vi "BeamScanner.vi"() -> ()   [LabVIEW 2016]
uses:
  C:/Program Files/Ocean Optics/OmniDriver/OOI_HOME/NETOmniDriver-NET40.dll
  Program Files/Ocean Optics/OmniDriver/OOI_HOME/NETOmniDriver-NET40.dll
  <vilib>/DAQmx/write.llb/DAQmx Write (Digital Bool 1Line 1Point).vi
  <vilib>/DAQmx/write.llb/DAQmx Write (Analog DBL 1Chan 1Samp).vi
  <vilib>/DAQmx/write.llb/DAQmx Write (Analog 1D DBL NChan 1Samp).vi
  <vilib>/DAQmx/write.llb/DAQmx Write (Analog 2D DBL NChan NSamp).vi
  <vilib>/Analysis/baseanly.llb/Mean (DBL).vi
  <vilib>/DAQmx/read.llb/DAQmx Read (Raw 1D I16).vi
  <vilib>/Analysis/1siggen.llb/Ramp Pattern by Samples.vi
  <vilib>/DAQmx/create/channels.llb/DAQmx Create Channel (DO-Digital Output).vi
  <vilib>/DAQmx/miscellaneous.llb/DAQmx Fill In Error Info.vi
  <vilib>/DAQmx/create/channels.llb/DAQmx Create Channel (AO-Voltage-Basic).vi
  resources/MotorPosition.vi
  <vilib>/DAQmx/create/channels.llb/DAQmx Create Channel (AI-Voltage-Basic).vi
  <vilib>/DAQmx/configure/timing.llb/DAQmx Timing (Sample Clock).vi
  <vilib>/DAQmx/configure/trigger.llb/DAQmx Start Trigger (Digital Edge).vi
  OCM/private/global.vi
  resources/xy_stack_global.vi
  <vilib>/Analysis/NI_AALBase.lvlib
  <resource>/objmgr/daqmx.rc
panel:
  out "Laser Blocking":string
  in  "Background":bool
  out "floor(x/y)":i32
  in  "Scan no.":i32
  in  "XY-Stack setup":bool
  in  "xy-Stacking":bool
  out "OCM Settings":T1
  out "Processed FFT":cluster{dbl[], "X":dbl[]}(graph)
  in  "length":i32=50
  in  "FFT index":i32=10
  out "OCM Array":dbl[][][](array[numeric])
  out "error out 2":errorcluster
  out "error out":errorcluster
  in  "OCM Setup":bool
  in  "Home X":dbl=-115.0
  in  "Home  Y":dbl=-88.0
  in  "sampling rate (ADC)":u32(ring)=1250000 items=["500000"=500000, "750000"=750000, "1000000"=1000000, "1250000"=1250000]
  in  "Intgration time [us]":u32=44444 min=100 max=10000000 step=1
  in  "Wavelength max":dbl=761.0 min=200.0 max=1100.0 step=1.0
  in  "Wavelength min":dbl=374.0 min=200.0 max=1100.0 step=1.0 format="%#.4g"
  out "spectral image":u32[][][](array[numeric])
  out "read task":refnum<k21>
  out "write task":refnum<k21>
  in  "Detector":u16(ring) items=["PMT", "QEPro", "Basler OCM", "Basler Confocal"]
  out "scanning waveforms":dbl[][](array[numeric])
  out "Retrace":dbl[][](array[numeric])
  in  "Move to z":bool
  out "z-Position":sgl format="%.2g"
  out "xy-Position [µm]":sgl[](array[numeric]) min=0 max=500
  in  "Thrown samples":i16=500
  in  "Throw away":bool
  out "Samples/Pixel":u32
  in  "PMT output range":dbl(ring)=0.1 items=["-0,1V – 0,1V"=0.1, "-0,2V – 0,2V"=0.2, "-0,5V – 0,5V"=0.5, "-1V – 1V"=1.0, "-2V – 2V"=2.0, "-5V – 5V"=5.0, "-10V – 10V"=10.0]
  out "Time of last scan memory":string
  out "Info File contents memory":string
  out "Info File contents":string
  out "Time per line [s]":dbl format="%#.1g"
  out "Time of last scan":string
  out "scaling factor (length/voltage)":dbl=228.9
  in  "Additional info":string
  in  "Save":bool
  in  "Quit":bool
  in  "PMT sensitivity":dbl min=-1989.12 max=1989.12 format="%#.2f"
  in  "requested z-Position":dbl min=0.0 max=10.0
  in  "# steps":u16=20 step=1 format="%#.0f"
  out "Duration (m.s)":string
  in  "Scanrate (pixels/s)":u32(ring)=10000 items=["250 kHz"=250000, "125 kHz"=125000, "50 kHz (!)"=50000, "25 kHz (!)"=25000, "10 kHz (?)"=10000, "5 kHz (?)"=5000, "2 kHz"=2000, "1 kHz"=1000, "500 Hz"=500, "200 Hz"=200, "100 Hz"=100]
  out "Optimal":string
  out "Optimal pixel size [nm]":dbl format="%#.0f"
  in  "NA":dbl=1.0 min=0.0
  in  "Swap Memory":bool
  out "Memory":dbl[][](graph)
  out "System":bool
  in  "Use white point":bool
  in  "Magnification":dbl=20.0
  in  "Go home":bool
  in  "Go to white point":bool
  in  "z-Maximum val":dbl min=0.0 max=500.0 format="%#.2f"
  in  "z-Minimum val":dbl min=0.0 max=500.0 format="%#.2f"
  in  "z-Stacking":bool
  in  "Step size":dbl=1.0 min=0.0
  in  "z-Minimum":dbl(slide) min=0.0 max=500.0 step=1.0 scale=0.0..500.0
  in  "z-Maximum":dbl(slide)=0.30612244897959184 min=370.0 max=500.0 step=1.0 scale=0.0..500.0
  out "Path":path
  in  "File identifier":string="unnamed_file"
  in  "Save Image":bool
  in  "Scan":bool
  in  "y-Offset":dbl=-160.0 min=-448.0 max=448.0 format="%#.2f"
  in  "x-Offset":dbl=-220.0 min=-448.0 max=448.0 format="%#.2f"
  in  "Field of View":dbl(ring)=0.471281296023564 items=["4x4 µm"=0.01747106355099367, "8x8 µm"=0.03494212710198734, "16x16 µm"=0.06988425420397468, "32x32 µm"=0.13976850840794935, "64x64 µm"=0.2795370168158987, "128x128 µm"=0.5590740336317974, "256x256 µm"=1.1181480672635948, "512x512 µm"=2.2362961345271897, "1024x1024 µm"=4.472592269054379, "0x0"=0.0]
  out "Image":dbl[][](graph)
  in  "Number of pixels":i32(ring)=128 items=["8x8"=8, "16x16"=16, "32x32"=32, "64x64"=64, "128x128"=128, "256x256"=256, "512x512"=512, "1024x1024"=1024, "optimal"=1280]
  # "OCM debugging"
  # "make setup button"
  # "MIN 7000 for QEPro"
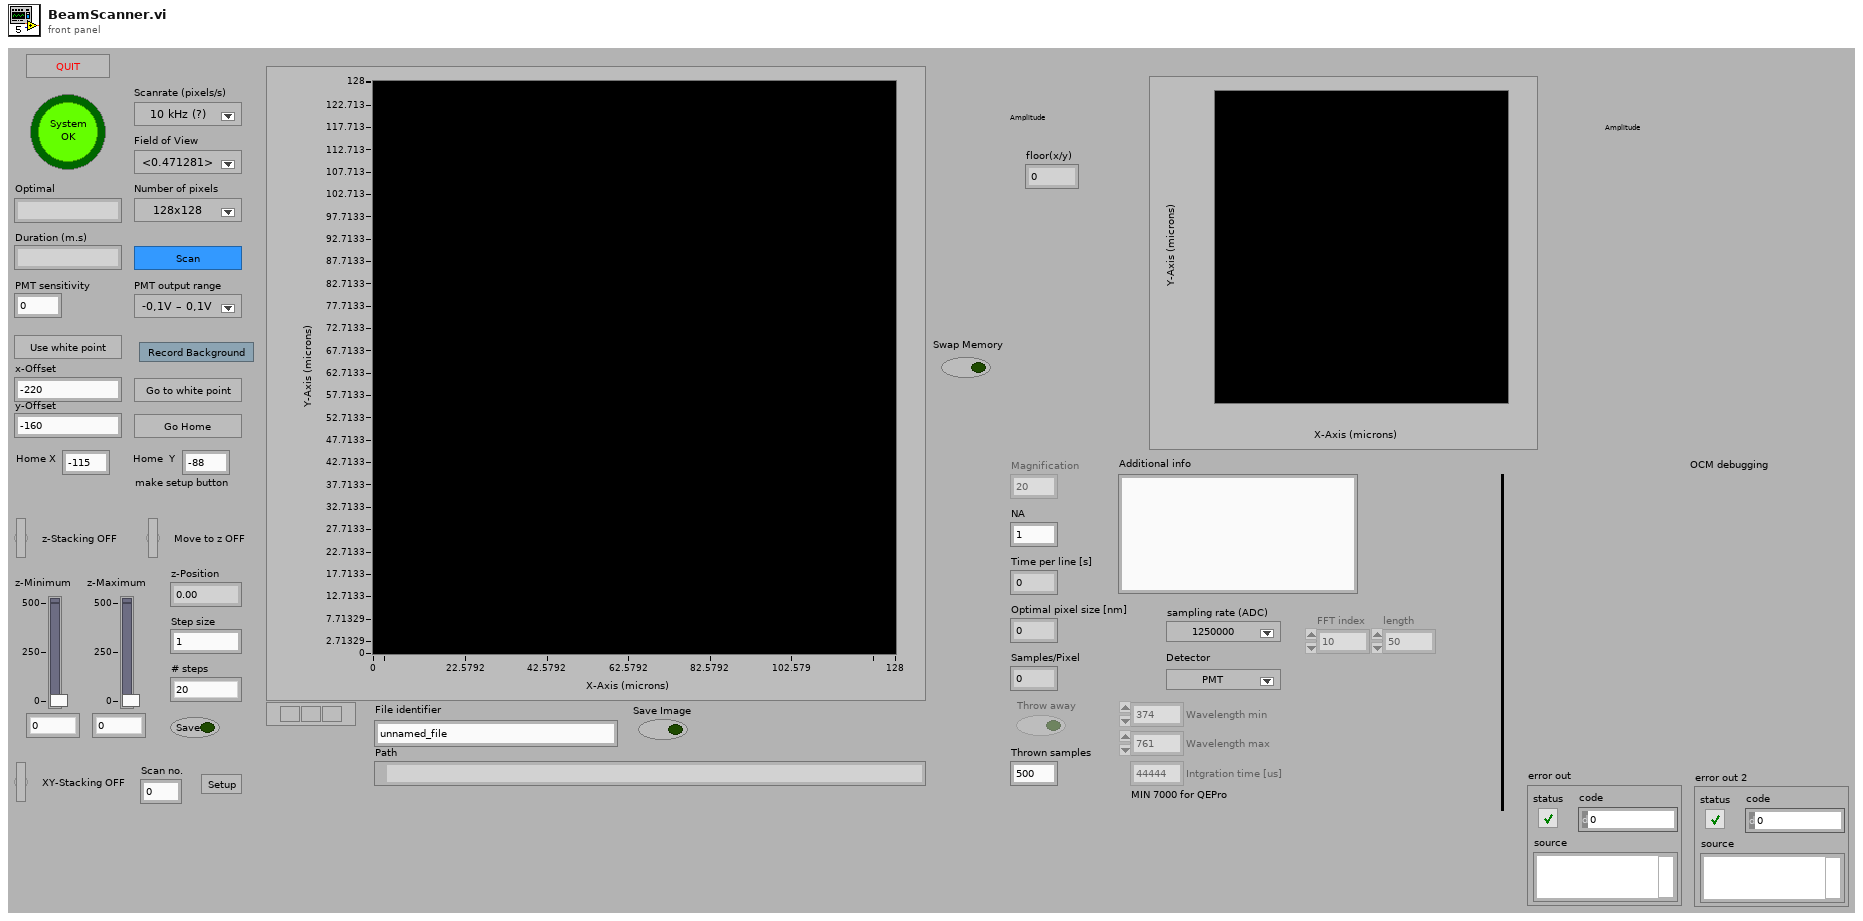
[diagram p1: front panel]
types:
  T1 = cluster{"Binning be4 FFT ":bool, "Pixels FFT":i32, "Camera averaging":bool, "FFT averaging":bool, "FFT AVG Size":dbl, "BG subtraction":bool, "DC compensation":bool, "BG Array":dbl[], "DC Array":dbl[], "k-array":dbl[], "axial distance array":dbl[], "k-ramp":dbl[]}
  T2 = enum8{"Enabled", "Disabled", "Disabled and Grayed Out"}
  T3 = enum32{"Invalid", "Standard", "Closed", "Hidden", "Minimized", "Maximized"}
  T4 = typedef "LVStringsAndValuesArrayTypeDef_DBL.ctl" = cluster{"String":string, "Value":dbl}[]
  T5 = typedef "LVStringsAndValuesArrayTypeDef_I32.ctl" = cluster{"String":string, "Value":i32}[]
  T6 = typedef "LVOffsetAndMultiplierTypeDef.ctl" = cluster{"Offset":dbl, "Multiplier":dbl}
  T7 = typedef "Maya2000 basic info.ctl" = cluster{"This instruments index":i32, "Name+SerialNumber":string, "Number Dark pixels":i32, "NumberOfPixels\nper spectrum":i32, "NumberOf Maya2000 instrm.":i32, "MaximumIntegrationTime\n[us]":i32, "MinimumIntegrationTime\n[us]":i32}
  T8 = typedef "IMAQ Image.ctl" = refnum<image>
  T9 = cluster{"Ramp Pattern":dbl[], "FFT Processed":dbl[]}
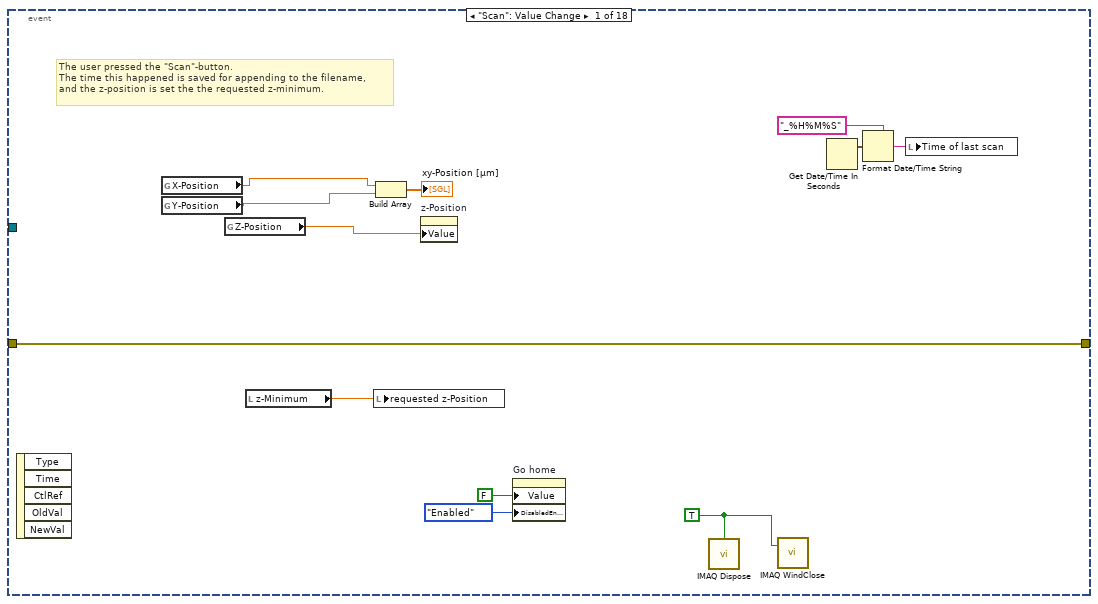
[diagram p3: hidden frame]
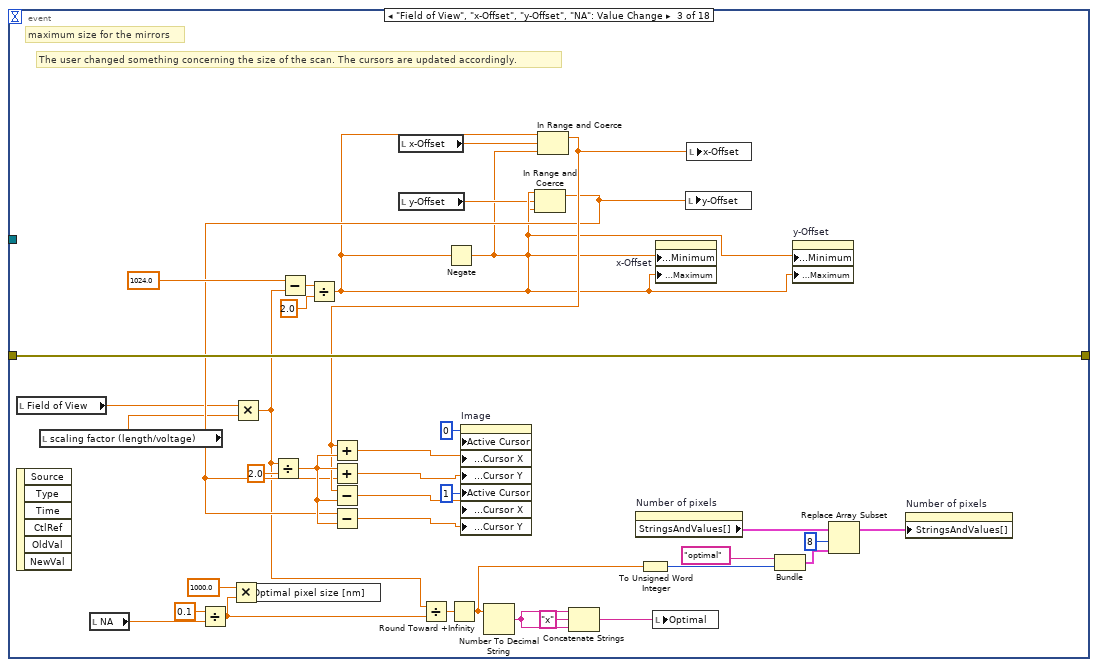
[diagram p5: hidden frame]
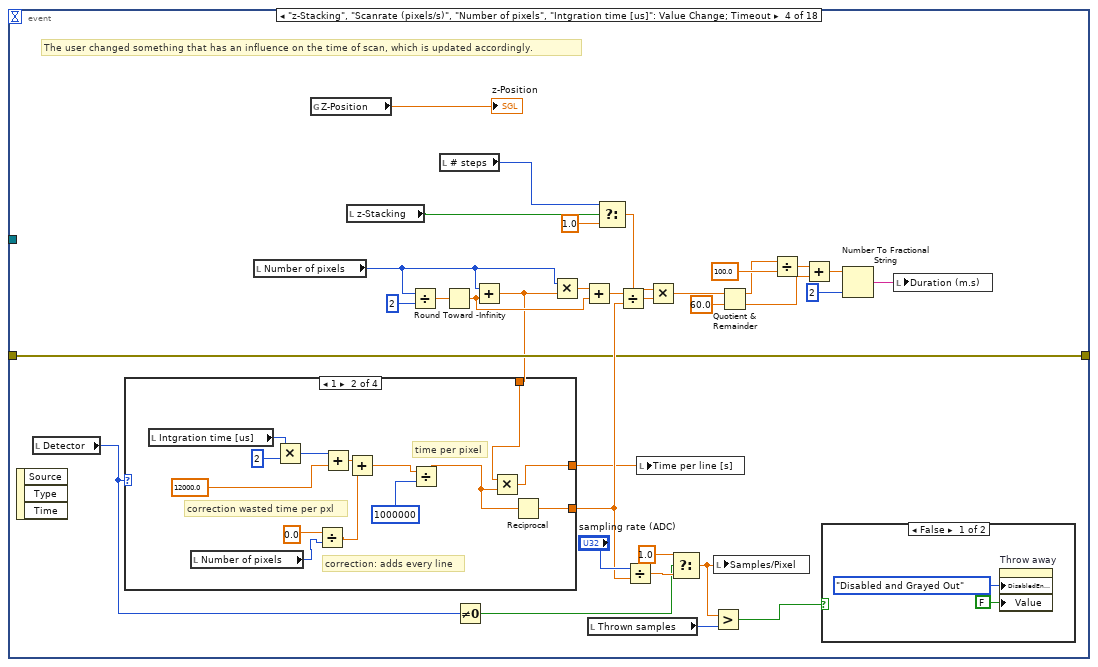
[diagram p6: hidden frame]
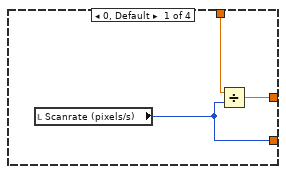
[diagram p7: hidden frame]
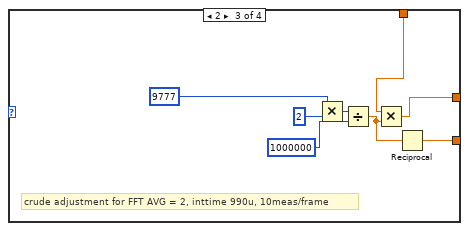
[diagram p8: hidden frame]
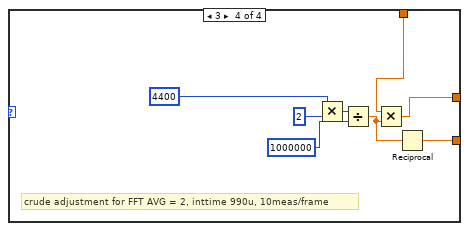
[diagram p9: hidden frame]
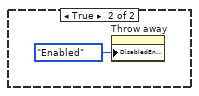
[diagram p10: hidden frame]
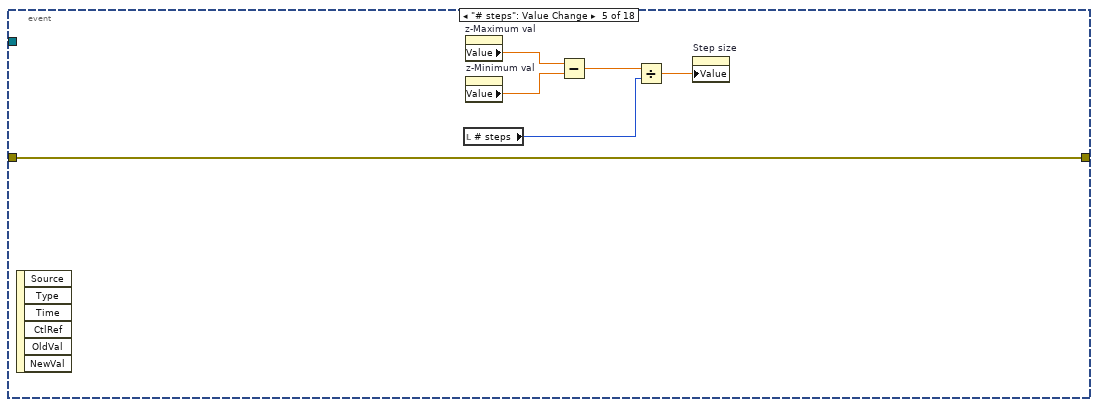
[diagram p11: hidden frame]
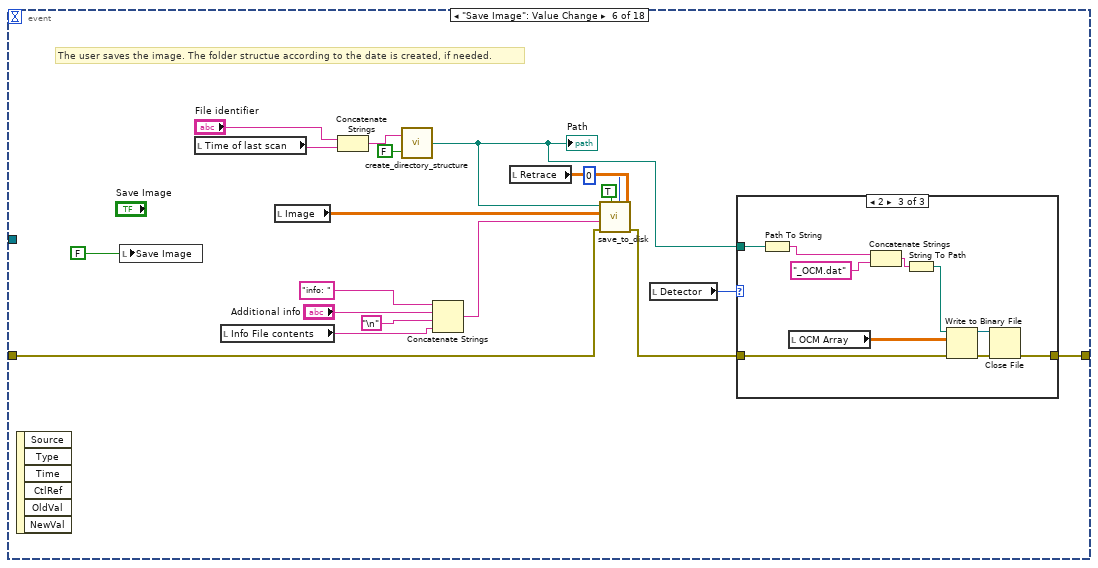
[diagram p12: hidden frame]
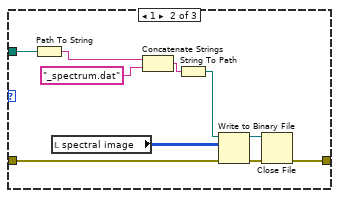
[diagram p14: hidden frame]
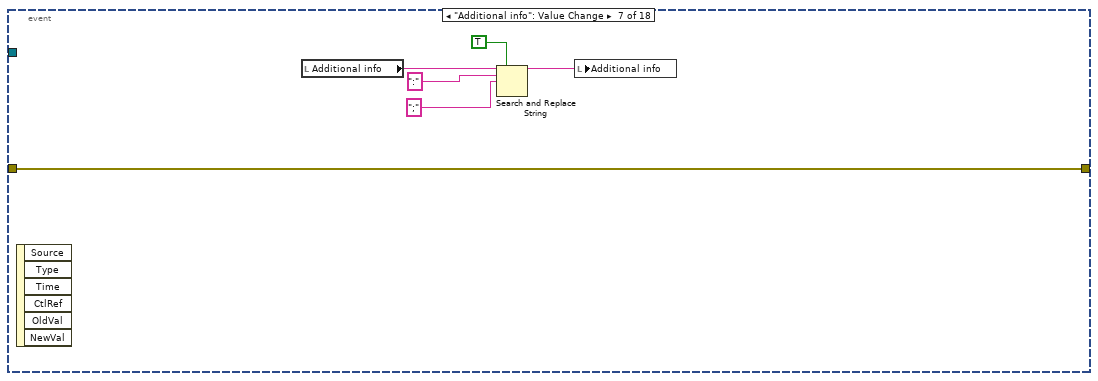
[diagram p15: hidden frame]
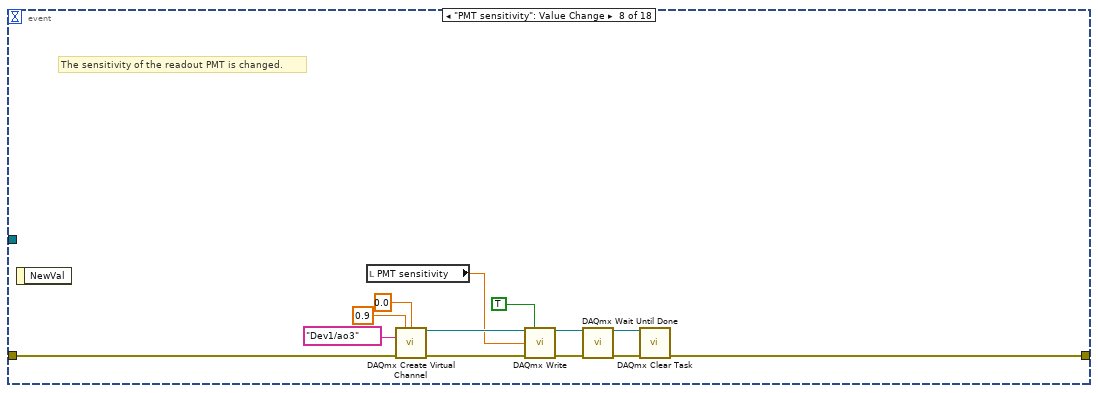
[diagram p16: hidden frame]
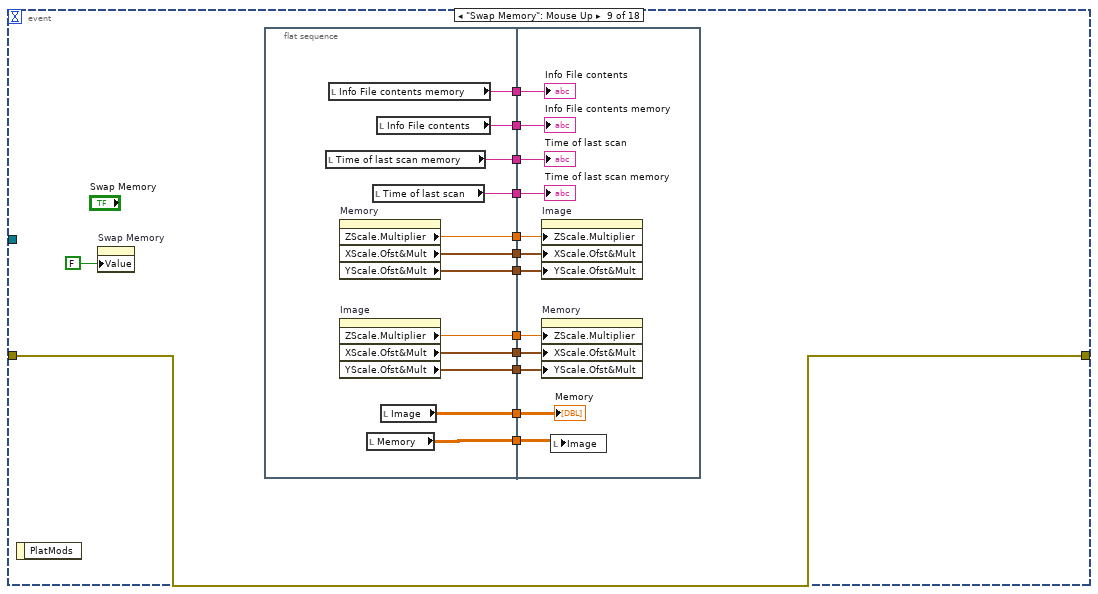
[diagram p17: hidden frame]
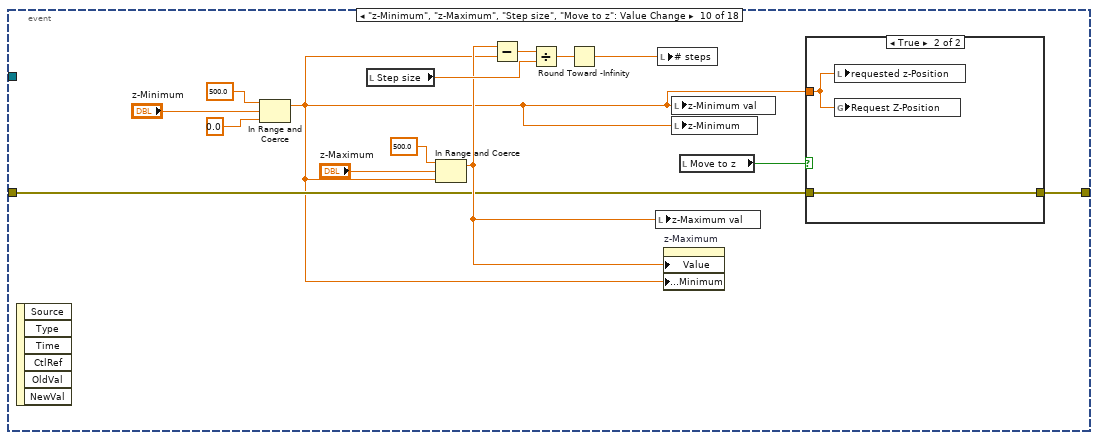
[diagram p18: hidden frame]
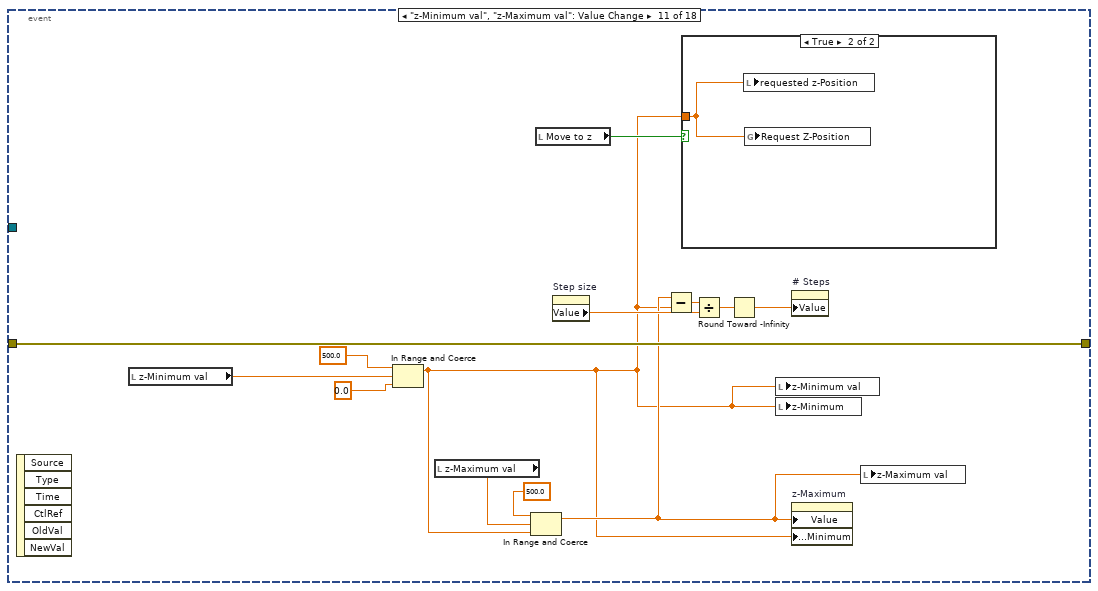
[diagram p20: hidden frame]
diagram:
  w1 = FALSE ("Visible")
  w15 = FALSE ("System")
  # "These are local variable containers,\ninvisible to the user"
  # "Close the shutter"
  # "First, we initialise a few values, e.g.\nthe \"Save Image\" button is hidden,\nand the \"Scan\" button is set to false."
  n1 = local read "Home  Y"() -> (w2:dbl)
  n2 = local read "Home X"() -> (w3:dbl)
  n3 = call-poly <vilib>:"DAQmx Create Virtual Channel.vi"("lines"=tag "Dev1/port2/line0") -> ("task out"=w63:refnum<k21>, "error out"=w62:errorcluster)  [unwired: 13 in]
  n4 = property on="System" class="Bool (strict)"("Value"=TRUE ("System")) -> ()  [unwired: 2 in, 2 out]
  n5 = property on="Go to white point" class="Bool (strict)"("Value"=w15) -> ()  [unwired: 2 in, 2 out]
  n6 = property on="Quit" class="Bool (strict)"("Value"=w15) -> ()  [unwired: 2 in, 2 out]
  n7 = property on="Scan" class="Bool (strict)"("Value"=w15) -> ()  [unwired: 2 in, 2 out]
  n8 = property on="Go home" class="Bool (strict)"("Value"=w15, "DisabledEnum"=T2."Enabled" ("Disabled")) -> ()  [unwired: 2 in, 2 out]
  n9 = local write "x-Offset"(w3) -> ()
  n10 = local write "y-Offset"(w2) -> ()
  n11 = property on="OCM Setup" class="Bool"("Visible"=FALSE) -> ()  [unwired: 2 in, 2 out]
  n12 = call-poly <vilib>:"DAQmx Write.vi"("task/channels in"=w63, "data"=FALSE, "error in"=w62) -> ("task out"=w60:refnum<k21>, "error out"=w59:errorcluster)  [unwired: 10 in, 1 out]
  n13 = property on="Magnification" class="DigNum (strict)"("DisabledEnum"=T2."Disabled and Grayed Out" ("Disabled")) -> ()  [unwired: 2 in, 2 out]
  n14 = call <vilib>:"DAQmx Clear Task.vi"("task in"=w60, "error in"=w59) -> ("error out"=w47:errorcluster)  [unwired: 13 in]
  n15 = property on="write task" class="DAQmxName (strict)"("Visible"=w1) -> ()  [unwired: 2 in, 2 out]
  n16 = property on="read task" class="DAQmxName (strict)"("Visible"=w1) -> ()  [unwired: 2 in, 2 out]
  n17 = property on="scanning waveforms" class="Arr (strict)"("Visible"=w1) -> ()  [unwired: 2 in, 2 out]
  n18 = property on="Retrace" class="Arr (strict)"("Visible"=w1) -> ()  [unwired: 2 in, 2 out]
  n19 = property on="info file contents" class="Str"("Visible"=w1) -> ()  [unwired: 2 in, 2 out]
  n20 = property on="time of last scan" class="Str"("Visible"=w1) -> ()  [unwired: 2 in, 2 out]
  n21 = property on="info file contents memory" class="Str"("Visible"=w1) -> ()  [unwired: 2 in, 2 out]
  n22 = property on="time of last scan memory" class="Str"("Visible"=w1) -> ()  [unwired: 2 in, 2 out]
  n23 = property on="scaling factor (length/voltage)" class="DigNum (strict)"("Visible"=w1) -> ()  [unwired: 2 in, 2 out]
  n24 = property on="xy-Position [µm]" class="Arr (strict)"("Visible"=w1) -> ()  [unwired: 2 in, 2 out]
  n25 = property on="spectral image" class="Arr (strict)"("Visible"=w1) -> ()  [unwired: 2 in, 2 out]
  n26 = property on="requested z-Position" class="DigNum (strict)"("Visible"=w1) -> ()  [unwired: 2 in, 2 out]
  n27 = property on="OCM Array" class="Arr (strict)"("Visible"=w1) -> ()  [unwired: 2 in, 2 out]
  n28 = property on="Laser Blocking" class="Str"("Visible"=w1) -> ()  [unwired: 2 in, 2 out]
  n29 = property on="OCM Settings" class="Clust (strict)"("Visible"=w1) -> ()  [unwired: 2 in, 2 out]
  n30 = Divide(x=0.1, y="NA") -> (x/y=w36:dbl)
  n31 = call-poly <vilib>:"DAQmx Create Virtual Channel.vi"("maximum value"=0.9, "minimum value"=0.0, "physical channels"=tag "Dev1/ao3", "error in"=w47) -> ("task out"=w51:refnum<k21>, "error out"=w50:errorcluster)  [unwired: 10 in]
  n32 = Divide(x=4301.0, y="Magnification") -> (x/y=w22:dbl)
  "scaling factor (length/voltage)" <- w22
  n33 = Multiply(x=1000.0, y=w36) -> (x*y=→"Optimal pixel size [nm]":dbl)
  n34 = call-poly <vilib>:"DAQmx Write.vi"("task/channels in"=w51, "auto start"=TRUE, "data"="PMT sensitivity", "error in"=w50) -> ("task out"=w54:refnum<k21>, "error out"=w53:errorcluster)  [unwired: 9 in, 1 out]
  n35 = for {
    N: 8 -> [_]
    tunnel: [w78] -> w30 mode=indexing
    i -> [w85]
    n36 = Add(x=3, y=w85) -> (x+y=w82:i32)
    n37 = Scale By Power Of 2(n=w82, x=u16 1) -> (x*2^n=w79:u16)
    n38 = Format Into String(format string="%dx%d", w79, w79) -> (resulting string=w80:string)  [unwired: 2 in, 1 out]
    n39 = Bundle(w80, w79) -> (w78:cluster{string, u16})  [unwired: 1 in]
  }
  n40 = call <vilib>:"DAQmx Wait Until Done.vi"("task/channels in"=w54, "error in"=w53) -> ("task out"=w49:refnum<k21>, "error out"=w48:errorcluster)  [unwired: 12 in]
  n41 = Multiply(x=w22, y="Field of View") -> (x*y=w40:dbl)
  n42 = call <vilib>:"DAQmx Clear Task.vi"("task in"=w49, "error in"=w48) -> ("error out"=w46:errorcluster)  [unwired: 13 in]
  n43 = Divide(x=w40, y=w36) -> (x/y=w39:dbl)
  n44 = Build Array(tag "Dev1/ao0" ("physical channels"), tag "Dev1/ao1" ("physical channels")) -> (w75:tag[])
  n45 = Round Toward +Infinity(x=w39) -> (ceil(x): smallest int >= x=w32:dbl)
  n46 = call <vilib>:"DAQmx Flatten Channel String.vi"("names in"=w75, "error in"=w46) -> ("names out"=w74:string, "error out"=w73:errorcluster)  [unwired: 12 in]
  n47 = Number To Decimal String(number=w32) -> (decimal integer string=w37:string)  [unwired: 1 in]
  n48 = To Unsigned Word Integer(number=w32) -> (unsigned 16bit integer=w31:u16)
  n49 = call-poly <vilib>:"DAQmx Create Virtual Channel.vi"("physical channels"=w74, "error in"=w73) -> ("task out"=w71:refnum<k21>, "error out"=w70:errorcluster)  [unwired: 12 in]
  n50 = for {
    N: 9 -> [_]
    tunnel: w22 -> [w88]
    tunnel: [w87] -> w20 mode=indexing
    i -> [w92]
    n51 = Add(x=2, y=w92) -> (x+y=w94:i32)
    n52 = Scale By Power Of 2(n=w94, x=u16 1) -> (x*2^n=w89:u16)
    n53 = Divide(x=w89, y=w88) -> (x/y=w86:dbl)
    n54 = Format Into String(format string="%dx%d \\B5m", w89, w89) -> (resulting string=w90:string)  [unwired: 2 in, 1 out]
    n55 = Bundle(w90, w86) -> (w87:cluster{string, dbl})  [unwired: 1 in]
  }
  n56 = Concatenate Strings(w37, "x" ("string"), w37) -> (→"Optimal":string)
  n57 = call-poly <vilib>:"DAQmx Write.vi"("task/channels in"=w71, "data"=dbl[] [0.0, 0.0], "error in"=w70) -> ("task out"=w68:refnum<k21>, "error out"=w66:errorcluster)  [unwired: 10 in, 1 out]
  n58 = Bundle("string"="optimal", w31) -> (w29:cluster{"string":string, u16})  [unwired: 1 in]
  n59 = call <vilib>:"DAQmx Wait Until Done.vi"("task/channels in"=w68, "error in"=w66) -> ("task out"=w67:refnum<k21>, "error out"=w65:errorcluster)  [unwired: 12 in]
  n60 = Build Array (concatenate)(w30, w29) -> (w28:cluster{"string":string, u16}[])
  n61 = call <vilib>:"DAQmx Clear Task.vi"("task in"=w67, "error in"=w65) -> ("error out"=w7:errorcluster)  [unwired: 13 in]
  n62 = property on="Number of pixels" class="Ring (strict)"("StringsAndValues[]"=w28) -> ()  [unwired: 2 in, 2 out]
  n63 = Open VI Reference(vi path=path "kinesis/kinesis.vi", error in (no error)=w7) -> (vi reference=w13:refnum<vi>, error out=w12:errorcluster)  [unwired: 4 in]
  n64 = invoke class="VI" method="Run VI"(reference=w13, error in=w12, "Wait until done"=FALSE ("Wait Until Done")) -> (reference out=w10:refnum<vi>, error out=w9:errorcluster)  [unwired: 2 in, 3 out]
  n65 = Bundle("format string"="0x0", 0.0) -> (w19:cluster{"format string":string, dbl})  [unwired: 1 in]
  n66 = Build Array (concatenate)(w20, w19) -> (w16:cluster{"format string":string, dbl}[])
  n67 = property on="Field of View" class="Ring (strict)"("Strings And Values []"=w16) -> ()  [unwired: 2 in, 2 out]
  n68 = invoke class="VI" method="FP.Open"(reference=w10, error in=w9, "Activate"=TRUE ("Activate?")) -> (reference out=w5:refnum<vi>, error out=w6:errorcluster)  [unwired: 2 in, 3 out]
  n69 = while {
    shift-right: [w98] -> w21
    shift-left: w6 -> [w104]
    tunnel: w5 -> [w96]
    stop <- w99 stop-if-true
    n70 = flat-sequence {
      tunnel: w104 -> [w108]
      tunnel: [w107] -> w105
      tunnel: w96 -> [w106]
      tunnel: w105 -> [w568]
      tunnel: [w568] -> w103
      tunnel: w103 -> [w616]
      tunnel: [w615] -> w102
      tunnel: w102 -> [w636]
      tunnel: [w635] -> w97
      tunnel: [w727] -> w101
      tunnel: [w726] -> w100
      tunnel: w97 -> [w725]
      tunnel: w101 -> [w1430]
      tunnel: w100 -> [w1427]
      tunnel: [w1428] -> w98
      tunnel: [w1431] -> w99
      frame #0 {
        n71 = while {
          shift-right: [w116] -> w107
          shift-left: w108 -> [w118]
          tunnel: w106 -> [w113]
          stop <- w112 stop-if-true
          # "The individual routines are called via events. The program waits, until an event occurs."
          n72 = event shown="[1] \"Image\": Cursor Release" {
            selector: _ -> [_ _ _ _ _ _ _ _ _ _ _ _ _ _ _ _ _ _]
            dyn-events: _ -> [_ _ _ _ _ _ _ _ _ _ _ _ _ _ _ _ _ _]
            timeout: 100 -> [_ _ _ _ _ _ _ _ _ _ _ _ _ _ _ _ _ _]
            tunnel: w118 -> [w125 w153 w212 w235 w295 w307 w341 w349 w364 w400 w421 w438 w455 w470 w485 _ _ w518]
            tunnel: [w125 w153 w212 w235 w295 w303 w341 w348 w364 w399 w421 w437 w454 w470 w485 w505 w510 w519] -> w116
            tunnel: w113 -> [_ _ _ _ _ _ _ _ _ _ _ _ _ _ _ _ _ w516]
            event "Scan": Value Change {
              w124 = TRUE ("All Images? (No)")
              # "The user pressed the \"Scan\"-button.\nThe time this happened is saved for appending to the filename,\nand the z-position is set the the requested z-minimum."
              n73 = event-data() -> ()  [unwired: 1 in, 5 out]
              n74 = global read "MotorPosition.vi" "X-Position"() -> (w121:dbl)
              n75 = global read "MotorPosition.vi" "Y-Position"() -> (w120:dbl)
              n76 = global read "MotorPosition.vi" "Z-Position"() -> (w123:dbl)
              n77 = local read "z-Minimum"() -> (w126:dbl)
              n78 = local write "requested z-Position"(w126) -> ()
              n79 = Build Array(w121, w120) -> (→"xy-Position [µm]":dbl[])
              n80 = property on="z-Position" class="DigNum (strict)"("Value"=w123) -> ()  [unwired: 2 in, 2 out]
              n81 = property on="Go home" class="Bool (strict)"("Value"=FALSE ("Go home"), "DisabledEnum"=T2."Enabled" ("Disabled")) -> ()  [unwired: 2 in, 2 out]
              n82 = call "IMAQ Dispose"("All Images? (No)"=w124) -> ()  [unwired: 5 in, 1 out]
              n83 = call "IMAQ WindClose"("Close All Windows (False)"=w124) -> ()  [unwired: 5 in, 1 out]
              n84 = Get Date/Time In Seconds() -> (seconds since 1Jan1904=w130:timestamp)
              n85 = Format Date/Time String(time format string (%c)="_%H%M%S", seconds (now)=w130) -> (date/time string=w127:string)  [unwired: 1 in]
              n86 = local write "Time of last scan"(w127) -> ()
            }
            event "Image": Cursor Release {
              w154 = 512.0 ("upper limit")
              w155 = -512.0 ("upper limit")
              # "The user moved a cursor in the graph.\nThe cursors are cropped, if necessary, for lying within the permissible area."
              n87 = event-data() -> ("CursIdx"=w133:i32)  [unwired: 1 in]
              n88 = property on="Image" class="IntGraph (strict)"("Active Cursor"=u32 0, "Active Cursor"=u32 1, "Active Cursor"=u32 2) -> ("Cursor.Cursor Position:Cursor X"=w152:dbl, "Cursor.Cursor Position:Cursor Y"=w151:dbl, "Cursor.Cursor Position:Cursor X"=w150:dbl, "Cursor.Cursor Position:Cursor Y"=w149:dbl, "Cursor.Cursor Position:Cursor X"=w148:dbl, "Cursor.Cursor Position:Cursor Y"=w147:dbl)  [unwired: 2 in, 2 out]
              n89 = Subtract(x=w152, y=w150) -> (x-y=w168:dbl)
              n90 = Max & Min(x=w152, y=w150) -> (min(x,y)=w165:dbl)  [unwired: 1 out]
              n91 = Absolute Value(x=w168) -> (abs(x)=w145:dbl)
              n92 = Subtract(x=w151, y=w149) -> (x-y=w167:dbl)
              n93 = Max & Min(x=w151, y=w149) -> (min(x,y)=w164:dbl)  [unwired: 1 out]
              n94 = Absolute Value(x=w167) -> (abs(x)=w146:dbl)
              n95 = Max & Min(x=w146, y=w145) -> (min(x,y)=w135:dbl)  [unwired: 1 out]
              n96 = Divide(x=w135, y=2.0) -> (x/y=w136:dbl)
              n97 = Add(x=w165, y=w136) -> (x+y=w144:dbl)
              n98 = Add(x=w164, y=w136) -> (x+y=w137:dbl)
              n99 = property on="x-Offset" class="DigNum (strict)"("Val(Sgnl)"=w144) -> ()  [unwired: 2 in, 2 out]
              n100 = local write "y-Offset"(w137) -> ()
              n101 = Not Equal?(x=w133, y=2) -> (x != y?=w134:bool)
              n102 = case shown="True" w134 {
                tunnel: w135 -> [_ w177]
                frame False {
                  # "The user moved the white cursor, so no updating is required"
                }
                frame True {
                  n103 = local read "Optimal pixel size [nm]"() -> (w181:dbl)
                  n104 = local read "scaling factor (length/voltage)"() -> (w180:dbl)
                  n105 = property on="Field of View" class="Ring (strict)"() -> ("StringsAndValues[]"=w176:T4)  [unwired: 2 in, 2 out]
                  n106 = Number To Decimal String(number=w177) -> (decimal integer string=w178:string)  [unwired: 1 in]
                  n107 = Divide(x=w177, y=w180) -> (x/y=w171:dbl)
                  n108 = Concatenate Strings(w178, "x" ("string"), w178) -> (w173:string)
                  n109 = Divide(x=w181, y=1000.0 ("x")) -> (x/y=w184:dbl)
                  n110 = Bundle(w173, w171) -> (w175:cluster{string, dbl})  [unwired: 1 in]
                  n111 = Divide(x=w177, y=w184) -> (x/y=w188:dbl)
                  n112 = Round Toward +Infinity(x=w188) -> (ceil(x): smallest int >= x=w187:dbl)
                  n113 = Number To Decimal String(number=w187) -> (decimal integer string=w185:string)  [unwired: 1 in]
                  n114 = Replace Array Subset(array=w176, new element=w175, index=9) -> (w172:T4)
                  n115 = Concatenate Strings(w185, "x" ("string"), w185) -> (w183:string)
                  n116 = property on="Field of View" class="Ring (strict)"("Value"=w171, "StringsAndValues[]"=w172) -> ()  [unwired: 2 in, 2 out]
                  n117 = local write "Optimal"(w183) -> ()
                }
              }
              n118 = Add(x=w137, y=w136) -> (x+y=w160:dbl)
              n119 = Subtract(x=w144, y=w136) -> (x-y=w159:dbl)
              n120 = Subtract(x=w137, y=w136) -> (x-y=w158:dbl)
              n121 = Add(x=w144, y=w136) -> (x+y=w161:dbl)
              n122 = In Range and Coerce(upper limit=w154, x=w161, lower limit=w155) -> (coerced(x)=w143:dbl)  [unwired: 1 out]
              n123 = In Range and Coerce(upper limit=w154, x=w160, lower limit=w155) -> (coerced(x)=w142:dbl)  [unwired: 1 out]
              n124 = In Range and Coerce(upper limit=w154, x=w159, lower limit=w155) -> (coerced(x)=w141:dbl)  [unwired: 1 out]
              n125 = In Range and Coerce(upper limit=w154, x=w158, lower limit=w155) -> (coerced(x)=w140:dbl)  [unwired: 1 out]
              n126 = In Range and Coerce(upper limit=w154, x=w148, lower limit=w155) -> (coerced(x)=w139:dbl)  [unwired: 1 out]
              n127 = In Range and Coerce(upper limit=w154, x=w147, lower limit=w155) -> (coerced(x)=w138:dbl)  [unwired: 1 out]
              n128 = property on="Image" class="IntGraph (strict)"("Active Cursor"=u32 0, "Cursor.Cursor Position:Cursor X"=w143, "Cursor.Cursor Position:Cursor Y"=w142, "Active Cursor"=u32 1, "Cursor.Cursor Position:Cursor X"=w141, "Cursor.Cursor Position:Cursor Y"=w140, "Active Cursor"=u32 2, "Cursor.Cursor Position:Cursor X"=w139, "Cursor.Cursor Position:Cursor Y"=w138) -> ()  [unwired: 2 in, 2 out]
            }
            event "Field of View", "x-Offset", "y-Offset", "NA": Value Change {
              # "The user changed something concerning the size of the scan. The cursors are updated accordingly."
              # "maximum size for the mirrors"
              n129 = local read "Field of View"() -> (w190:dbl)
              n130 = event-data() -> ()  [unwired: 1 in, 6 out]
              n131 = local read "scaling factor (length/voltage)"() -> (w194:dbl)
              n132 = local read "NA"() -> (w211:dbl)
              n133 = Divide(x=0.1, y=w211) -> (x/y=w214:dbl)
              n134 = Multiply(x=1000.0, y=w214) -> (x*y=w210:dbl)
              n135 = Multiply(x=w190, y=w194) -> (x*y=w189:dbl)
              n136 = local write "Optimal pixel size [nm]"(w210) -> ()
              n137 = Divide(x=w189, y=2.0) -> (x/y=w225:dbl)
              n138 = Subtract(x=1024.0, y=w189) -> (x-y=w220:dbl)
              n139 = Divide(x=w220, y=2.0) -> (x/y=w195:dbl)
              n140 = local read "x-Offset"() -> (w193:dbl)
              n141 = local read "y-Offset"() -> (w192:dbl)
              n142 = Divide(x=w189, y=w214) -> (x/y=w217:dbl)
              n143 = Negate(x=w195) -> (-x=w191:dbl)
              n144 = Round Toward +Infinity(x=w217) -> (ceil(x): smallest int >= x=w208:dbl)
              n145 = Number To Decimal String(number=w208) -> (decimal integer string=w215:string)  [unwired: 1 in]
              n146 = In Range and Coerce(upper limit=w195, x=w192, lower limit=w191) -> (coerced(x)=w200:dbl)  [unwired: 1 out]
              n147 = Add(x=w225, y=w200) -> (x+y=w198:dbl)
              n148 = Subtract(x=w200, y=w225) -> (x-y=w196:dbl)
              n149 = In Range and Coerce(upper limit=w195, x=w193, lower limit=w191) -> (coerced(x)=w201:dbl)  [unwired: 1 out]
              n150 = Add(x=w201, y=w225) -> (x+y=w199:dbl)
              n151 = Subtract(x=w201, y=w225) -> (x-y=w197:dbl)
              n152 = property on="Image" class="IntGraph (strict)"("Active Cursor"=u32 0, "Cursor.Cursor Position:Cursor X"=w199, "Cursor.Cursor Position:Cursor Y"=w198, "Active Cursor"=u32 1, "Cursor.Cursor Position:Cursor X"=w197, "Cursor.Cursor Position:Cursor Y"=w196) -> ()  [unwired: 2 in, 2 out]
              n153 = Concatenate Strings(w215, "x" ("string"), w215) -> (w207:string)
              n154 = property on="Number of pixels" class="Ring (strict)"() -> ("StringsAndValues[]"=w204:T5)  [unwired: 2 in, 2 out]
              n155 = To Unsigned Word Integer(number=w208) -> (unsigned 16bit integer=w209:u16)
              n156 = local write "Optimal"(w207) -> ()
              n157 = property on="x-Offset" class="DigNum (strict)"("Data Range:Minimum"=w191, "Data Range:Maximum"=w195) -> ()  [unwired: 2 in, 2 out]
              n158 = local write "y-Offset"(w200) -> ()
              n159 = local write "x-Offset"(w201) -> ()
              n160 = Bundle("string"="optimal", w209) -> (w206:cluster{"string":string, u16})  [unwired: 1 in]
              n161 = property on="y-Offset" class="DigNum (strict)"("Data Range:Minimum"=w191, "Data Range:Maximum"=w195) -> ()  [unwired: 2 in, 2 out]
              n162 = Replace Array Subset(array=w204, new element=w206, index=8) -> (w205:T5)
              n163 = property on="Number of pixels" class="Ring (strict)"("StringsAndValues[]"=w205) -> ()  [unwired: 2 in, 2 out]
            }
            event "z-Stacking", "Scanrate (pixels/s)", "Number of pixels", "Intgration time [us]": Value Change; Timeout {
              # "The user changed something that has an influence on the time of scan, which is updated accordingly."
              n164 = event-data() -> ()  [unwired: 1 in, 3 out]
              n165 = local read "Detector"() -> (w229:u16)
              n166 = local read "Number of pixels"() -> (w234:i32)
              n167 = global read "MotorPosition.vi" "Z-Position"() -> (→"z-Position":dbl)
              n168 = local read "z-Stacking"() -> (w240:bool)
              n169 = Divide(x=w234, y=2) -> (x/y=w258:dbl)
              n170 = local read "# steps"() -> (w243:u16)
              n171 = Round Toward -Infinity(1:w258) -> (0:w256:dbl)
              n172 = Not Equal To 0?(x=w229) -> (x != 0?=w228:bool)
              n173 = Add(x=w234, y=w256) -> (x+y=w233:dbl)
              n174 = case shown="1" w229 {
                tunnel: [w261 w274 w281 w289] -> w238
                tunnel: w233 -> [w260 w275 w282 w290]
                tunnel: [w259 w273 w280 w288] -> w227
                frame 0, Default {
                  n175 = local read "Scanrate (pixels/s)"() -> (w261:u32)
                  n176 = Divide(x=w260, y=w261) -> (x/y=w259:dbl)
                }
                frame 1 {
                  # "correction wasted time per pxl"
                  # "correction: adds every line"
                  # "time per pixel"
                  n177 = local read "Intgration time [us]"() -> (w272:u32)
                  n178 = local read "Number of pixels"() -> (w263:i32)
                  n179 = Multiply(x=w272, y=u32 2) -> (x*y=w268:u32)
                  n180 = Divide(x=0.0, y=w263) -> (x/y=w262:dbl)
                  n181 = Add(x=w268, y=12000.0) -> (x+y=w270:dbl)
                  n182 = Add(x=w270, y=w262) -> (x+y=w266:dbl)
                  n183 = Divide(x=w266, y=u32 1000000) -> (x/y=w267:dbl)
                  n184 = Multiply(x=w275, y=w267) -> (x*y=w273:dbl)
                  n185 = Reciprocal(x=w267) -> (1/x=w274:dbl)
                }
                frame 2 {
                  # "crude adjustment for FFT AVG = 2, inttime 990u, 10meas/frame"
                  n186 = Multiply(x=u32 9777, y=u32 2) -> (x*y=w278:u32)
                  n187 = Divide(x=w278, y=u32 1000000) -> (x/y=w279:dbl)
                  n188 = Multiply(x=w282, y=w279) -> (x*y=w280:dbl)
                  n189 = Reciprocal(x=w279) -> (1/x=w281:dbl)
                }
                frame 3 {
                  # "crude adjustment for FFT AVG = 2, inttime 990u, 10meas/frame"
                  n190 = Multiply(x=u32 4400, y=u32 2) -> (x*y=w286:u32)
                  n191 = Divide(x=w286, y=u32 1000000) -> (x/y=w287:dbl)
                  n192 = Multiply(x=w290, y=w287) -> (x*y=w288:dbl)
                  n193 = Reciprocal(x=w287) -> (1/x=w289:dbl)
                }
              }
              n194 = Multiply(x=w234, y=w233) -> (x*y=w257:dbl)
              n195 = Add(x=w257, y=w256) -> (x+y=w255:dbl)
              n196 = local read "Thrown samples"() -> (w236:i16)
              n197 = Select(t=w243, s=w240, f=1.0) -> (s? t:f=w252:dbl)
              n198 = Divide(x=w255, y=w238) -> (x/y=w253:dbl)
              n199 = Divide(x="sampling rate (ADC)", y=w238) -> (x/y=w232:dbl)
              n200 = local write "Time per line [s]"(w227) -> ()
              n201 = Multiply(x=w252, y=w253) -> (x*y=w246:dbl)
              n202 = Select(t=1.0, s=w228, f=w232) -> (s? t:f=w231:dbl)
              n203 = Greater?(x=w231, y=w236) -> (0:w237:bool)
              n204 = local write "Samples/Pixel"(w231) -> ()
              n205 = Quotient & Remainder(x=w246, y=60.0) -> (x-y*floor(x/y)=w244:dbl, floor(x/y)=w250:dbl)
              n206 = Divide(x=w244, y=100.0) -> (x/y=w245:dbl)
              n207 = Add(x=w245, y=w250) -> (x+y=w248:dbl)
              n208 = case shown="False" w237 {
                frame False {
                  n209 = property on="Throw away" class="Bool (strict)"("DisabledEnum"=T2."Disabled and Grayed Out" ("Disabled"), "Value"=FALSE ("Throw away")) -> ()  [unwired: 2 in, 2 out]
                }
                frame True {
                  n210 = property on="Throw away" class="Bool (strict)"("DisabledEnum"=T2."Enabled" ("Disabled")) -> ()  [unwired: 2 in, 2 out]
                }
              }
              n211 = Number To Fractional String(number=w248, precision (6)=i16 2) -> (F-format string=w242:string)  [unwired: 2 in]
              n212 = local write "Duration (m.s)"(w242) -> ()
            }
            event "# steps": Value Change {
              n213 = event-data() -> ()  [unwired: 1 in, 6 out]
              n214 = local read "# steps"() -> (w296:u16)
              n215 = property on="z-Maximum val" class="DigNum (strict)"() -> ("Value"=w300:dbl)  [unwired: 2 in, 2 out]
              n216 = property on="z-Minimum val" class="DigNum (strict)"() -> ("Value"=w299:dbl)  [unwired: 2 in, 2 out]
              n217 = Subtract(x=w300, y=w299) -> (x-y=w298:dbl)
              n218 = Divide(x=w298, y=w296) -> (x/y=w297:dbl)
              n219 = property on="Step size" class="DigNum (strict)"("Value"=w297) -> ()  [unwired: 2 in, 2 out]
            }
            event "Save Image": Value Change {
              # "The user saves the image. The folder structue according to the date is created, if needed."
              n220 = event-data() -> ()  [unwired: 1 in, 6 out]
              n221 = local write "Save Image"(FALSE ("Bild speichern ...")) -> ()
              n222 = local read "Time of last scan"() -> (w318:string)
              n223 = local read "Info File contents"() -> (w311:string)
              n224 = local read "Image"() -> (w316:dbl[][])
              n225 = Concatenate Strings("File identifier", w318) -> (w310:string)
              n226 = call "create_directory_structure.vi"("Z-stack"=FALSE, "File identifier"=w310) -> ("File path"=w304:path)
              "Path" <- w304
              n227 = Concatenate Strings("info: " ("format string"), "Additional info", "\n", w311) -> (w315:string)
              n228 = local read "Retrace"() -> (w308:dbl[][])
              n229 = call "save_to_disk.vi"("Retrace"=w308, "slice"=0, "write info file?"=TRUE, "error in"=w307, "Scan info"=w315, "Image"=w316, "File path"=w304) -> ("error out"=w305:errorcluster)  [unwired: 2 in]
              n230 = local read "Detector"() -> (w302:u16)
              n231 = case shown="2" w302 {
                tunnel: w305 -> [w320 w329 w339]
                tunnel: w304 -> [_ w328 w338]
                tunnel: [w320 w321 w331] -> w303
                frame 0, Default {
                }
                frame 1 {
                  n232 = Path To String(path=w328) -> (string=w325:string)
                  n233 = local read "spectral image"() -> (w330:u32[][][])
                  n234 = Concatenate Strings(w325, "_spectrum.dat" ("string")) -> (w327:string)
                  n235 = String To Path(string=w327) -> (path=w324:path)
                  n236 = Write to Binary File(file (use dialog)=w324, data=w330, error in=w329) -> (refnum out=w322:refnum<file>, error out=w323:errorcluster)  [unwired: 3 in, 1 out]
                  n237 = Close File(refnum=w322, error in=w323) -> (error out=w321:errorcluster)  [unwired: 1 out]
                }
                frame 2 {
                  n238 = Path To String(path=w338) -> (string=w335:string)
                  n239 = local read "OCM Array"() -> (w340:dbl[][][])
                  n240 = Concatenate Strings(w335, "_OCM.dat" ("string")) -> (w337:string)
                  n241 = String To Path(string=w337) -> (path=w334:path)
                  n242 = Write to Binary File(file (use dialog)=w334, data=w340, error in=w339) -> (refnum out=w332:refnum<file>, error out=w333:errorcluster)  [unwired: 3 in, 1 out]
                  n243 = Close File(refnum=w332, error in=w333) -> (error out=w331:errorcluster)  [unwired: 1 out]
                }
              }
            }
            event "Additional info": Value Change {
              n244 = event-data() -> ()  [unwired: 1 in, 6 out]
              n245 = local read "Additional info"() -> (w342:string)
              n246 = Search and Replace String(replace all?=TRUE ("replace all? (F)"), input string=w342, search string=":", replace string=";") -> (result string=w343:string)  [unwired: 4 in, 3 out]
              n247 = local write "Additional info"(w343) -> ()
            }
            event "PMT sensitivity": Value Change {
              # "The sensitivity of the readout PMT is changed."
              n248 = event-data() -> ()  [unwired: 1 in, 1 out]
              n249 = local read "PMT sensitivity"() -> (w347:dbl)
              n250 = call-poly <vilib>:"DAQmx Create Virtual Channel.vi"("maximum value"=0.9, "minimum value"=0.0, "physical channels"=tag "Dev1/ao3", "error in"=w349) -> ("task out"=w353:refnum<k21>, "error out"=w352:errorcluster)  [unwired: 10 in]
              n251 = call-poly <vilib>:"DAQmx Write.vi"("task/channels in"=w353, "auto start"=TRUE, "data"=w347, "error in"=w352) -> ("task out"=w356:refnum<k21>, "error out"=w355:errorcluster)  [unwired: 9 in, 1 out]
              n252 = call <vilib>:"DAQmx Wait Until Done.vi"("task/channels in"=w356, "error in"=w355) -> ("task out"=w351:refnum<k21>, "error out"=w350:errorcluster)  [unwired: 12 in]
              n253 = call <vilib>:"DAQmx Clear Task.vi"("task in"=w351, "error in"=w350) -> ("error out"=w348:errorcluster)  [unwired: 13 in]
            }
            event "Swap Memory": Mouse Up {
              n254 = event-data() -> ()  [unwired: 1 in, 1 out]
              n255 = property on="Swap Memory" class="Bool (strict)"("Value"=FALSE ("Swap Memory")) -> ()  [unwired: 2 in, 2 out]
              n256 = flat-sequence {
                tunnel: [w385] -> w372
                tunnel: [w384] -> w371
                tunnel: [w383] -> w370
                tunnel: [w382] -> w369
                tunnel: [w381] -> w368
                tunnel: [w380] -> w367
                tunnel: [w379] -> w366
                tunnel: [w378] -> w365
                tunnel: [w377] -> w363
                tunnel: [w376] -> w362
                tunnel: [w375] -> w361
                tunnel: [w374] -> w360
                tunnel: w372 -> [w391]
                tunnel: w371 -> [w397]
                tunnel: w370 -> [w390]
                tunnel: w369 -> [w396]
                tunnel: w368 -> [w395]
                tunnel: w367 -> [w394]
                tunnel: w366 -> [w393]
                tunnel: w365 -> [w392]
                tunnel: w363 -> [w389]
                tunnel: w362 -> [w388]
                tunnel: w361 -> [w387]
                tunnel: w360 -> [w386]
                frame #0 {
                  n257 = local read "Time of last scan memory"() -> (w383:string)
                  n258 = local read "Info File contents memory"() -> (w385:string)
                  n259 = property on="Memory" class="IntGraph (strict)"() -> ("ZScale.Multiplier"=w381:dbl, "XScale.Ofst&Mult"=w377:T6, "YScale.Ofst&Mult"=w376:T6)  [unwired: 2 in, 2 out]
                  n260 = property on="Image" class="IntGraph (strict)"() -> ("ZScale.Multiplier"=w380:dbl, "XScale.Ofst&Mult"=w375:T6, "YScale.Ofst&Mult"=w374:T6)  [unwired: 2 in, 2 out]
                  n261 = local read "Memory"() -> (w379:dbl[][])
                  n262 = local read "Time of last scan"() -> (w382:string)
                  n263 = local read "Info File contents"() -> (w384:string)
                  n264 = local read "Image"() -> (w378:dbl[][])
                }
                frame #1 {
                  n265 = property on="Image" class="IntGraph (strict)"("ZScale.Multiplier"=w395, "XScale.Ofst&Mult"=w389, "YScale.Ofst&Mult"=w388) -> ()  [unwired: 2 in, 2 out]
                  n266 = property on="Memory" class="IntGraph (strict)"("ZScale.Multiplier"=w394, "XScale.Ofst&Mult"=w387, "YScale.Ofst&Mult"=w386) -> ()  [unwired: 2 in, 2 out]
                  n267 = local write "Image"(w393) -> ()
                  "Info File contents memory" <- w397
                  "Time of last scan memory" <- w396
                  "Memory" <- w392
                  "Info File contents" <- w391
                  "Time of last scan" <- w390
                }
              }
            }
            event "z-Minimum", "z-Maximum", "Step size", "Move to z": Value Change {
              n268 = event-data() -> ()  [unwired: 1 in, 6 out]
              n269 = In Range and Coerce(upper limit=500.0, x="z-Minimum", lower limit=0.0) -> (coerced(x)=w398:dbl)  [unwired: 1 out]
              n270 = local read "Step size"() -> (w404:dbl)
              n271 = In Range and Coerce(upper limit=500.0, x="z-Maximum", lower limit=w398) -> (coerced(x)=w402:dbl)  [unwired: 1 out]
              n272 = Subtract(x=w402, y=w398) -> (x-y=w407:dbl)
              n273 = Divide(x=w407, y=w404) -> (x/y=w406:dbl)
              n274 = Round Toward -Infinity(1:w406) -> (0:w405:dbl)
              n275 = local write "z-Maximum val"(w402) -> ()
              n276 = local write "# steps"(w405) -> ()
              n277 = property on="z-Maximum" class="Slide (strict)"("Value"=w402, "Data Range:Minimum"=w398) -> ()  [unwired: 2 in, 2 out]
              n278 = local write "z-Minimum val"(w398) -> ()
              n279 = local write "z-Minimum"(w398) -> ()
              n280 = local read "Move to z"() -> (w401:bool)
              n281 = case shown="True" w401 {
                tunnel: w400 -> [w412 w414]
                tunnel: [w412 w414] -> w399
                tunnel: w398 -> [_ w413]
                frame False {
                }
                frame True {
                  n282 = local write "requested z-Position"(w413) -> ()
                  n283 = global write "MotorPosition.vi" "Request Z-Position"(w413) -> ()
                }
              }
            }
            event "z-Minimum val", "z-Maximum val": Value Change {
              n284 = event-data() -> ()  [unwired: 1 in, 6 out]
              n285 = local read "z-Minimum val"() -> (w420:dbl)
              n286 = In Range and Coerce(upper limit=500.0, x=w420, lower limit=0.0) -> (coerced(x)=w415:dbl)  [unwired: 1 out]
              n287 = local read "z-Maximum val"() -> (w419:dbl)
              n288 = In Range and Coerce(upper limit=500.0, x=w419, lower limit=w415) -> (coerced(x)=w417:dbl)  [unwired: 1 out]
              n289 = local read "Move to z"() -> (w416:bool)
              n290 = property on="Step size" class="DigNum (strict)"() -> ("Value"=w424:dbl)  [unwired: 2 in, 2 out]
              n291 = Subtract(x=w417, y=w415) -> (x-y=w425:dbl)
              n292 = case shown="True" w416 {
                tunnel: w415 -> [_ w428]
                frame False {
                }
                frame True {
                  n293 = local write "requested z-Position"(w428) -> ()
                  n294 = global write "MotorPosition.vi" "Request Z-Position"(w428) -> ()
                }
              }
              n295 = Divide(x=w425, y=w424) -> (x/y=w423:dbl)
              n296 = Round Toward -Infinity(1:w423) -> (0:w422:dbl)
              n297 = local write "z-Minimum val"(w415) -> ()
              n298 = local write "z-Minimum"(w415) -> ()
              n299 = property on="# Steps" class="DigNum (strict)"("Value"=w422) -> ()  [unwired: 2 in, 2 out]
              n300 = property on="z-Maximum" class="Slide (strict)"("Value"=w417, "Data Range:Minimum"=w415) -> ()  [unwired: 2 in, 2 out]
              n301 = local write "z-Maximum val"(w417) -> ()
            }
            event "Go to white point": Value Change {
              w442 = FALSE ("Go to black point")
              n302 = event-data() -> ()  [unwired: 1 in, 6 out]
              n303 = local read "scaling factor (length/voltage)"() -> (w433:dbl)
              n304 = property on="Image" class="IntGraph (strict)"(error in=w438, "Active Cursor"=u32 2) -> (error out=w439:errorcluster, "Cursor.Cursor Position:Cursor X"=w432:dbl, "Cursor.Cursor Position:Cursor Y"=w430:dbl)  [unwired: 1 in, 1 out]
              n305 = Negate(x=w432) -> (-x=w431:dbl)
              n306 = Negate(x=w430) -> (-x=w429:dbl)
              n307 = Divide(x=w431, y=w433) -> (x/y=w435:dbl)
              n308 = Divide(x=w429, y=w433) -> (x/y=w436:dbl)
              n309 = Build Array(w435, w436) -> (w443:dbl[])
              n310 = call "go_to_point.vi"("error in"=w439, "data"=w443) -> ("error out"=w441:errorcluster)
              n311 = property on="Go to white point" class="Bool (strict)"(error in=w441, "Value"=w442) -> (error out=w440:errorcluster)  [unwired: 1 in, 1 out]
              n312 = property on="Go home" class="Bool (strict)"(error in=w440, "Value"=w442, "Disabled"=T2."Enabled") -> (error out=w437:errorcluster)  [unwired: 1 in, 1 out]
            }
            event "Go home": Value Change {
              n313 = event-data() -> ()  [unwired: 1 in, 6 out]
              n314 = local read "scaling factor (length/voltage)"() -> (w445:dbl)
              n315 = Negate(x="Home X") -> (-x=w448:dbl)
              n316 = Negate(x="Home  Y") -> (-x=w450:dbl)
              n317 = property on="Go home" class="Bool (strict)"("Disabled"=T2."Disabled") -> ()  [unwired: 2 in, 2 out]
              n318 = Divide(x=w448, y=w445) -> (x/y=w446:dbl)
              n319 = Divide(x=w450, y=w445) -> (x/y=w451:dbl)
              n320 = Build Array(w446, w451) -> (w452:dbl[])
              n321 = call "go_to_point.vi"("error in"=w455, "data"=w452) -> ("error out"=w454:errorcluster)
            }
            event "Use white point": Value Change {
              n322 = event-data() -> ()  [unwired: 1 in, 6 out]
              n323 = local read "scaling factor (length/voltage)"() -> (w464:dbl)
              n324 = local read "Field of View"() -> (w469:dbl)
              n325 = Multiply(x=w464, y=w469) -> (x*y=w465:dbl)
              n326 = flat-sequence {
                frame #0 {
                  n327 = Wait (ms)(milliseconds to wait=u32 250) -> ()  [unwired: 1 out]
                }
                frame #1 {
                  n328 = Not(x="Use white point") -> (.not. x?=w477:bool)
                  n329 = property on="Use white point" class="Bool (strict)"("Value"=w477) -> ()  [unwired: 2 in, 2 out]
                }
              }
              n330 = Divide(x=w465, y=2.0) -> (x/y=w456:dbl)
              n331 = property on="Image" class="IntGraph (strict)"("Active Cursor"=u32 2) -> ("Cursor.Cursor Position:Cursor X"=w467:dbl, "Cursor.Cursor Position:Cursor Y"=w466:dbl)  [unwired: 2 in, 2 out]
              n332 = Subtract(x=512.0, y=w456) -> (x-y=w463:dbl)
              n333 = Negate(x=w463) -> (-x=w462:dbl)
              n334 = In Range and Coerce(upper limit=w463, x=w466, lower limit=w462) -> (coerced(x)=w457:dbl)  [unwired: 1 out]
              n335 = In Range and Coerce(upper limit=w463, x=w467, lower limit=w462) -> (coerced(x)=w468:dbl)  [unwired: 1 out]
              n336 = property on="x-Offset" class="DigNum (strict)"("Data Range:Minimum"=w462, "Data Range:Maximum"=w463) -> ()  [unwired: 2 in, 2 out]
              n337 = property on="y-Offset" class="DigNum (strict)"("Data Range:Minimum"=w462, "Data Range:Maximum"=w463) -> ()  [unwired: 2 in, 2 out]
              n338 = local write "x-Offset"(w468) -> ()
              n339 = local write "y-Offset"(w457) -> ()
              n340 = Add(x=w468, y=w456) -> (x+y=w458:dbl)
              n341 = Add(x=w457, y=w456) -> (x+y=w459:dbl)
              n342 = Subtract(x=w468, y=w456) -> (x-y=w460:dbl)
              n343 = Subtract(x=w457, y=w456) -> (x-y=w461:dbl)
              n344 = property on="Image" class="IntGraph (strict)"("Active Cursor"=u32 0, "Cursor.Cursor Position:Cursor X"=w458, "Cursor.Cursor Position:Cursor Y"=w459, "Active Cursor"=u32 1, "Cursor.Cursor Position:Cursor X"=w460, "Cursor.Cursor Position:Cursor Y"=w461) -> ()  [unwired: 2 in, 2 out]
            }
            event "Detector": Value Change {
              n345 = event-data() -> ()  [unwired: 1 in, 6 out]
              n346 = local read "Detector"() -> (w483:u16)
              n347 = case shown="3" w483 {
                tunnel: [w487 w494 w499 w500] -> w486
                tunnel: [w490 T2."Enabled" ("Disabled") T2."Enabled" ("Disabled") T2."Enabled" ("Disabled")] -> w484
                tunnel: [w490 w494 w499 T2."Disabled and Grayed Out" ("Disabled")] -> w482
                tunnel: [FALSE TRUE FALSE FALSE] -> w480
                tunnel: [T2."Disabled and Grayed Out" ("Disabled") T2."Enabled" ("Disabled") w499 T2."Disabled and Grayed Out" ("Disabled")] -> w481
                tunnel: [w487 T2."Enabled" ("Disabled") T2."Enabled" ("Disabled") w500] -> w479
                frame 0, Default {
                  w487 = T2."Disabled and Grayed Out" ("Disabled")
                  w490 = T2."Enabled" ("Disabled")
                  # "PMT"
                }
                frame 2 {
                  w494 = T2."Disabled and Grayed Out" ("Disabled")
                  # "OCM"
                }
                frame 3 {
                  w499 = T2."Disabled and Grayed Out" ("Disabled")
                  # "Confocal"
                }
                frame 1 {
                  w500 = T2."Enabled" ("Disabled")
                  # "QEPRo"
                }
              }
              n348 = property on="FFT index" class="DigNum (strict)"("DisabledEnum"=w481) -> ()  [unwired: 2 in, 2 out]
              n349 = property on="length" class="DigNum (strict)"("DisabledEnum"=w481) -> ()  [unwired: 2 in, 2 out]
              n350 = property on="x-Offset" class="DigNum (strict)"("DisabledEnum"=w484) -> ()  [unwired: 2 in, 2 out]
              n351 = property on="y-Offset" class="DigNum (strict)"("DisabledEnum"=w484) -> ()  [unwired: 2 in, 2 out]
              n352 = property on="Use white point" class="Bool (strict)"("DisabledEnum"=w484) -> ()  [unwired: 2 in, 2 out]
              n353 = property on="Wavelength min" class="DigNum (strict)"("DisabledEnum"=w486) -> ()  [unwired: 2 in, 2 out]
              n354 = property on="Wavelength max" class="DigNum (strict)"("DisabledEnum"=w486) -> ()  [unwired: 2 in, 2 out]
              n355 = property on="Intgration time [us]" class="DigNum (strict)"("DisabledEnum"=w479) -> ()  [unwired: 2 in, 2 out]
              n356 = property on="PMT sensitivity" class="DigNum (strict)"("DisabledEnum"=w482) -> ()  [unwired: 2 in, 2 out]
              n357 = property on="PMT output range" class="Ring (strict)"("DisabledEnum"=w482) -> ()  [unwired: 2 in, 2 out]
              n358 = property on="Scanrate (pixels/s)" class="Ring (strict)"("DisabledEnum"=w482) -> ()  [unwired: 2 in, 2 out]
              n359 = property on="OCM Setup" class="Bool"("Visible"=w480) -> ()  [unwired: 2 in, 2 out]
              n360 = property on="Processed FFT" class="XYGraph (strict)"("Visible"=w480) -> ()  [unwired: 2 in, 2 out]
            }
            event "OCM Setup": Value Change {
              # "Open OCM Setup / Adjustment upon request"
              n361 = event-data() -> ()  [unwired: 1 in, 6 out]
              n362 = Open VI Reference(vi path=path "OCM/A-Scan.vi" ("Save Spectrum to: 2")) -> (vi reference=w508:refnum<vi>)  [unwired: 5 in, 1 out]
              n363 = invoke class="VI" method="FP.Open"(reference=w508, "Activate"=TRUE ("Activate?"), "State"=T3."Standard") -> (error out=w505:errorcluster)  [unwired: 2 in, 4 out]
            }
            event "XY-Stack setup": Value Change {
              # "Open OCM Setup / Adjustment upon request"
              n364 = event-data() -> ()  [unwired: 1 in, 6 out]
              n365 = Open VI Reference(vi path=path "resources/xy_stack_setup.vi" ("Save Spectrum to: 2")) -> (vi reference=w513:refnum<vi>)  [unwired: 5 in, 1 out]
              n366 = invoke class="VI" method="FP.Open"(reference=w513, "Activate"=TRUE ("Activate?"), "State"=T3."Standard") -> (error out=w510:errorcluster)  [unwired: 2 in, 4 out]
            }
            event "Quit": Mouse Down {
              n367 = event-data() -> ()  [unwired: 1 in, 8 out]
              n368 = flat-sequence {
                tunnel: w518 -> [w521]
                tunnel: [w521] -> w515
                tunnel: [w523] -> w517
                tunnel: w516 -> [w531]
                tunnel: w515 -> [w532]
                tunnel: [w544] -> w519
                tunnel: w517 -> [w544]
                frame #0 {
                  n369 = Wait (ms)(milliseconds to wait=u32 500) -> ()  [unwired: 1 out]
                }
                frame #1 {
                  n370 = call-poly <vilib>:"DAQmx Create Virtual Channel.vi"("maximum value"=0.75, "minimum value"=0.0, "physical channels"=tag "Dev1/ao3", "error in"=w532) -> ("task out"=w537:refnum<k21>, "error out"=w536:errorcluster)  [unwired: 10 in]
                  n371 = call-poly <vilib>:"DAQmx Write.vi"("task/channels in"=w537, "auto start"=TRUE, "data"=0.0, "error in"=w536) -> ("task out"=w540:refnum<k21>, "error out"=w539:errorcluster)  [unwired: 9 in, 1 out]
                  n372 = call <vilib>:"DAQmx Wait Until Done.vi"("task/channels in"=w540, "error in"=w539) -> ("task out"=w535:refnum<k21>, "error out"=w534:errorcluster)  [unwired: 12 in]
                  n373 = call <vilib>:"DAQmx Clear Task.vi"("task in"=w535, "error in"=w534) -> ("error out"=w530:errorcluster)  [unwired: 13 in]
                  n374 = invoke class="VI" method="FP.Close"(reference=w531, error in=w530) -> (reference out=w529:refnum<vi>, error out=w528:errorcluster)  [unwired: 1 in, 1 out]
                  n375 = invoke class="VI" method="Ctrl Val.Set"(reference=w529, error in=w528, "Control Name"="QUIT", "Value"=TRUE) -> (reference out=w525:refnum<vi>, error out=w524:errorcluster)  [unwired: 1 in, 3 out]
                  n376 = Close Reference(reference=w525, error in (no error)=w524) -> (error out=w523:errorcluster)
                  "error out" <- w523
                  n377 = Wait (ms)(milliseconds to wait=u32 500) -> ()  [unwired: 1 out]
                }
                frame #2 {
                  n378 = Stop() -> ()  [unwired: 1 in]
                  "error out 2" <- w544
                }
              }
            }
          }
          n379 = local read "Background"() -> (w110:bool)
          n380 = Unbundle By Name(w116) -> ("status"=w115:bool)
          "System" <- w115
          n381 = Not(x=w115) -> (.not. x?=w114:bool)
          n382 = And(x="Scan", y=w110) -> (x .and. y?=w109:bool)
          n383 = case shown="True" w109 {
            frame False {
            }
            frame True {
              n384 = property on="Laser Blocking" class="Str"("Visible"=TRUE) -> ()  [unwired: 2 in, 2 out]
            }
          }
          n385 = And(x=w114, y="Scan") -> (x .and. y?=w112:bool)
        }
      }
      frame #1 {
        # "These are the info-file contents"
        n386 = local read "Field of View"() -> (w573:dbl)
        n387 = local read "Number of pixels"() -> (w559:i32)
        n388 = Get Date/Time In Seconds() -> (seconds since 1Jan1904=w548:timestamp)
        n389 = local read "x-Offset"() -> (w550:dbl)
        n390 = local read "y-Offset"() -> (w558:dbl)
        n391 = local read "scaling factor (length/voltage)"() -> (w572:dbl)
        n392 = local read "Magnification"() -> (w560:dbl)
        n393 = local read "NA"() -> (w581:dbl)
        n394 = local read "Detector"() -> (w546:u16)
        n395 = local read "PMT sensitivity"() -> (w578:dbl)
        n396 = local read "PMT output range"() -> (w580:dbl)
        n397 = local read "PMT output range"() -> (w582:dbl)
        n398 = local read "Scanrate (pixels/s)"() -> (w579:u32)
        n399 = local read "z-Minimum"() -> (w577:dbl)
        n400 = local read "z-Stacking"() -> (w576:bool)
        n401 = local read "z-Maximum"() -> (w575:dbl)
        n402 = local read "Step size"() -> (w570:dbl)
        n403 = local read "# steps"() -> (w574:u16)
        n404 = local read "xy-Position [µm]"() -> (w567:sgl[])
        n405 = local read "Move to z"() -> (w561:bool)
        n406 = local read "z-Stacking"() -> (w553:bool)
        n407 = local read "Save"() -> (w552:bool)
        n408 = Format Date/Time String(time format string (%c)="%Y-%m-%d, %H%M%S", seconds (now)=w548) -> (date/time string=w547:string)  [unwired: 1 in]
        n409 = Boolean To (0,1)(Boolean=w576) -> (0, 1=w583:i16)
        n410 = Multiply(x=w573, y=w572) -> (x*y=w557:dbl)
        n411 = Not(x=w553) -> (.not. x?=w555:bool)
        n412 = Or(x=w561, y=w553) -> (x .or. y?=w556:bool)
        n413 = And(x=w553, y=w552) -> (x .and. y?=w551:bool)
        n414 = Boolean To (0,1)(Boolean=w555) -> (0, 1=w554:i16)
        n415 = Negate(x=w580) -> (-x=w571:dbl)
        n416 = case shown="True" w551 {
          frame False {
          }
          frame True {
            n417 = local read "File identifier"() -> (w586:string)
            n418 = local read "Time of last scan"() -> (w587:string)
            n419 = Concatenate Strings(w586, w587) -> (w588:string)
            n420 = call "create_directory_structure.vi"("Z-stack"=FALSE, "File identifier"=w588) -> ("File path"=w589:path)
            n421 = local write "Path"(w589) -> ()
          }
        }
        n422 = local write "Move to z"(w556) -> ()
        n423 = local write "# steps"(w554) -> ()
        n424 = Index Array(array=w567, index #1=0 ("index"), index #2=1 ("index")) -> (element #1=w564:sgl, element #2=w562:sgl)
        n425 = Boolean To (0,1)(Boolean=w556) -> (0, 1=w563:i16)
        n426 = local read "Intgration time [us]"() -> (w545:u32)
        n427 = Format Into String(format string="%.;%.;Date: %s\nx-offset: %f\ny-offset: %f\nImage Width: %f\nResolution: %d\nobj magn: %d\nNA: %f\nDetector Type: %f\nPMT sensitivity: %f\nDAQ readout min: %f\nDAQ readout max: %f\nScanrate (pixels/s): %d\nz-Minimum: %f\nz-stacking: %u\nz-Maximum: %f\nstep-value: %f\nnumber of steps: %d\nMotor x-pos [µm]: %f\nMotor y-pos [µm]: %f\nMove to z at scan: %u\nIntegration time [us]: %d\n", w547, w550, w558, w557, w559, w560, w581, w546, w578, w571, w582, w579, w577, w583, w575, w570, w574, w564, w562, w563, w545) -> (resulting string=w569:string)  [unwired: 2 in, 1 out]
        n428 = local write "Info File contents"(w569) -> ()
      }
      frame #2 {
        # "The waveforms for the two channels are created"
        n429 = local read "Number of pixels"() -> (w603:i32)
        n430 = local read "z-Stacking"() -> (w592:bool)
        n431 = local read "Save"() -> (w590:bool)
        n432 = Initialize Array(i16 0 ("element"), w603, w603) -> (w605:i16[][])
        n433 = Not(x=w590) -> (.not. x?=w591:bool)
        n434 = local read "scaling factor (length/voltage)"() -> (w610:dbl)
        n435 = local write "Image"(w605) -> ()
        n436 = Compound Arithmetic op=AND(w592, w591) -> (w593:bool)
        n437 = case shown="True" w593 {
          frame False {
          }
          frame True {
            n438 = One Button Dialog(message="Not saving!") -> ()  [unwired: 1 in, 1 out]
          }
        }
        n439 = call "createScanArrays.vi"("error in"=w616, "resolution"=w603) -> ("error out"=w615:errorcluster, "y-array"=w609:dbl[], "x-array"=w608:dbl[])  [unwired: 3 in]
        n440 = local read "Field of View"() -> (w602:dbl)
        n441 = local read "x-Offset"() -> (w611:dbl)
        n442 = local read "y-Offset"() -> (w598:dbl)
        n443 = Divide(x=w598, y=w610) -> (x/y=w596:dbl)
        n444 = Divide(x=w611, y=w610) -> (x/y=w595:dbl)
        n445 = Multiply(x=w608, y=w602) -> (x*y=w612:dbl[])
        n446 = Multiply(x=w609, y=w602) -> (x*y=w613:dbl[])
        n447 = Multiply(x=w602, y=w610) -> (x*y=w601:dbl)
        n448 = Divide(x=w601, y=2.0) -> (x/y=w597:dbl)
        n449 = Subtract(x=w612, y=w596) -> (x-y=w607:dbl[])
        n450 = Subtract(x=w613, y=w595) -> (x-y=w606:dbl[])
        n451 = Subtract(x=w611, y=w597) -> (x-y=w600:dbl)
        n452 = Subtract(x=w598, y=w597) -> (x-y=w599:dbl)
        n453 = Divide(x=w601, y=w603) -> (x/y=w614:dbl)
        n454 = Build Array(w607, w606) -> (→"scanning waveforms":dbl[][])
        n455 = property on="Image" class="IntGraph (strict)"("X Scale.Offset and Multiplier:Multiplier"=w614, "X Scale.Offset and Multiplier:Offset"=w600, "Y Scale.Offset and Multiplier:Multiplier"=w614, "Y Scale.Offset and Multiplier:Offset"=w599) -> (error out=w619:errorcluster)  [unwired: 2 in, 1 out]
        n456 = property on="Image" class="IntGraph (strict)"(error in=w619) -> ("X Scale.Range:Minimum"=w623:dbl, "Y Scale.Range:Minimum"=w622:dbl, "X Scale.Range:Maximum"=w621:dbl, "Y Scale.Range:Maximum"=w620:dbl)  [unwired: 1 in, 2 out]
        n457 = Subtract(x=w620, y=w622) -> (x-y=w627:dbl)
        n458 = Divide(x=w627, y=2.0) -> (x/y=w625:dbl)
        n459 = Add(x=w625, y=w622) -> (x+y=w624:dbl)
        n460 = Subtract(x=w621, y=w623) -> (x-y=w631:dbl)
        n461 = Divide(x=w631, y=2.0) -> (x/y=w628:dbl)
        n462 = Add(x=w628, y=w623) -> (x+y=w630:dbl)
        n463 = property on="Image" class="IntGraph (strict)"("Active Cursor"=u32 1, "Cursor.Cursor Position:Cursor X"=w623, "Cursor.Cursor Position:Cursor Y"=w622, "Active Cursor"=u32 0, "Cursor.Cursor Position:Cursor X"=w621, "Cursor.Cursor Position:Cursor Y"=w620, "Active Cursor"=u32 2, "Cursor.Cursor Position:Cursor X"=w630, "Cursor.Cursor Position:Cursor Y"=w624) -> ()  [unwired: 2 in, 2 out]
      }
      frame #3 {
        n464 = case shown="3" "Detector" {
          tunnel: [w654 w686 w700 w713] -> w635
          tunnel: w636 -> [w646 w687 w701 w714]
          frame 0, Default {
            w651 = 10348 items=["Volts"=10348, "From Custom Scale"=10065] ("units")
            w659 = 10348 items=["Volts"=10348, "From Custom Scale"=10065] ("units")
            w661 = 10083 items=["default"=-1, "RSE"=10083, "NRSE"=10078, "Differential"=10106, "Pseudodifferential"=12529] ("input terminal configuration")
            w673 = 10178 items=["Finite Samples"=10178, "Continuous Samples"=10123, "Hardware Timed Single Point"=12522] ("sample mode")
            # "Both the writing task (top) and the reading task (bottom) are initialised, but not started yet."
            n465 = local read "scanning waveforms"() -> (w641:dbl[][])
            n466 = Build Array(tag "Dev1/ao1" ("physical channels"), tag "Dev1/ao0" ("physical channels")) -> (w645:tag[])
            n467 = call <vilib>:"DAQmx Flatten Channel String.vi"("names in"=w645, "error in"=w646) -> ("names out"=w642:string, "error out"=w647:errorcluster)  [unwired: 12 in]
            n468 = Array Max & Min(array=w641) -> (max value=w644:dbl, min value=w643:dbl)  [unwired: 2 out]
            n469 = call-poly <vilib>:"DAQmx Create Virtual Channel.vi"("maximum value"=w644, "minimum value"=w643, "physical channels"=w642, "units"=w651, "error in"=w647) -> ("task out"=w648:refnum<k21>, "error out"=w649:errorcluster)  [unwired: 9 in]
            n470 = local read "PMT output range"() -> (w663:dbl)
            n471 = Array Size(array=w641) -> (size(s)=w667:i32[])
            n472 = Negate(x=w663) -> (-x=w662:dbl)
            n473 = local read "Samples/Pixel"() -> (w670:u32)
            n474 = call-poly <vilib>:"DAQmx Create Virtual Channel.vi"("maximum value"=w663, "minimum value"=w662, "input terminal configuration"=w661, "physical channels"=tag "Dev1/ai0", "units"=w659, "error in"=w649) -> ("task out"=w656:refnum<k21>)  [unwired: 8 in, 1 out]
            n475 = Index Array(array=w667, index=1) -> (element=w664:i32)
            n476 = Divide(x=w663, y=32767.0) -> (x/y=w657:dbl)
            n477 = Divide(x=w664, y=2) -> (x/y=w666:dbl)
            n478 = property on="Image" class="IntGraph (strict)"("ZScale.Multiplier"=w657) -> ()  [unwired: 2 in, 2 out]
            n479 = local read "Scanrate (pixels/s)"() -> (w684:u32)
            n480 = Multiply(x=w666, y=w670) -> (x*y=w672:dbl)
            n481 = local read "sampling rate (ADC)"() -> (w638:u32)
            n482 = Max & Min(x=w672, y=u32 25000000) -> (min(x,y)=w675:dbl)  [unwired: 1 out]
            n483 = call <vilib>:"DAQmx Configure Input Buffer.vi"("task/channels in"=w656, "buffer size (in samples per channel)"=w675) -> ("task out"=w682:refnum<k21>, "error out"=w676:errorcluster)  [unwired: 12 in]
            n484 = Multiply(x=w684, y=u32 2) -> (x*y=w669:u32)
            n485 = call-poly <vilib>:"DAQmx Timing.vi"("task/channels in"=w648, "sample mode"=w673, "samples per channel"=w664, "rate"=w669, "error in"=w649) -> ("task out"=w681:refnum<k21>, "error out"=w678:errorcluster)  [unwired: 9 in]
            n486 = call-poly <vilib>:"DAQmx Timing.vi"("task/channels in"=w682, "sample mode"=w673, "samples per channel"=w672, "rate"=w638, "error in"=w676) -> ("task out"=w683:refnum<k21>, "error out"=w674:errorcluster)  [unwired: 9 in]
            n487 = property class="DAQmx Read"(reference=w683, error in=w674, "Read All Available Samples"=TRUE ("ReadAllAvailSamp")) -> (reference out=→"read task":refnum<k21>, error out=w655:errorcluster)
            n488 = call-poly <vilib>:"DAQmx Trigger.vi"("task/channels in"=w681, "source"=tag "/Dev1/ai/StartTrigger", "error in"=w678) -> ("task out"=→"write task":refnum<k21>, "error out"=w639:errorcluster)  [unwired: 11 in]
            n489 = Merge Errors(w639, w655) -> (w654:errorcluster)
          }
          frame 1 {
            w695 = 10348 items=["Volts"=10348, "From Custom Scale"=10065] ("units")
            n490 = local read "scanning waveforms"() -> (w688:dbl[][])
            n491 = Build Array(tag "Dev1/ao1" ("physical channels"), tag "Dev1/ao0" ("physical channels")) -> (w692:tag[])
            n492 = call <vilib>:"DAQmx Flatten Channel String.vi"("names in"=w692, "error in"=w687) -> ("names out"=w689:string, "error out"=w693:errorcluster)  [unwired: 12 in]
            n493 = Array Max & Min(array=w688) -> (max value=w691:dbl, min value=w690:dbl)  [unwired: 2 out]
            n494 = call-poly <vilib>:"DAQmx Create Virtual Channel.vi"("maximum value"=w691, "minimum value"=w690, "physical channels"=w689, "units"=w695, "error in"=w693) -> ("task out"=w685:refnum<k21>, "error out"=w686:errorcluster)  [unwired: 9 in]
            n495 = local write "write task"(w685) -> ()
            n496 = property on="Image" class="IntGraph (strict)"("ZScale.Multiplier"=1.0 ("Z Scale.Offset and Multiplier:Multiplier")) -> ()  [unwired: 2 in, 2 out]
          }
          frame 2 {
            w709 = 10348 items=["Volts"=10348, "From Custom Scale"=10065] ("units")
            # "OCM copy&paste from QEPRO"
            n497 = local read "scanning waveforms"() -> (w702:dbl[][])
            n498 = property on="Image" class="IntGraph (strict)"("ZScale.Multiplier"=1.0 ("Z Scale.Offset and Multiplier:Multiplier")) -> ()  [unwired: 2 in, 2 out]
            n499 = Build Array(tag "Dev1/ao1" ("physical channels"), tag "Dev1/ao0" ("physical channels")) -> (w706:tag[])
            n500 = call <vilib>:"DAQmx Flatten Channel String.vi"("names in"=w706, "error in"=w701) -> ("names out"=w703:string, "error out"=w707:errorcluster)  [unwired: 12 in]
            n501 = Array Max & Min(array=w702) -> (max value=w705:dbl, min value=w704:dbl)  [unwired: 2 out]
            n502 = call-poly <vilib>:"DAQmx Create Virtual Channel.vi"("maximum value"=w705, "minimum value"=w704, "physical channels"=w703, "units"=w709, "error in"=w707) -> ("task out"=w699:refnum<k21>, "error out"=w700:errorcluster)  [unwired: 9 in]
            n503 = local write "write task"(w699) -> ()
            n504 = global read "global.vi" "OCM Settings"() -> (→"OCM Settings":T1)
          }
          frame 3 {
            w722 = 10348 items=["Volts"=10348, "From Custom Scale"=10065] ("units")
            # "Confocal copy&paste from QEPRO"
            n505 = local read "scanning waveforms"() -> (w715:dbl[][])
            n506 = property on="Image" class="IntGraph (strict)"("ZScale.Multiplier"=1.0 ("Z Scale.Offset and Multiplier:Multiplier")) -> ()  [unwired: 2 in, 2 out]
            n507 = Build Array(tag "Dev1/ao1" ("physical channels"), tag "Dev1/ao0" ("physical channels")) -> (w719:tag[])
            n508 = call <vilib>:"DAQmx Flatten Channel String.vi"("names in"=w719, "error in"=w714) -> ("names out"=w716:string, "error out"=w720:errorcluster)  [unwired: 12 in]
            n509 = Array Max & Min(array=w715) -> (max value=w718:dbl, min value=w717:dbl)  [unwired: 2 out]
            n510 = call-poly <vilib>:"DAQmx Create Virtual Channel.vi"("maximum value"=w718, "minimum value"=w717, "physical channels"=w716, "units"=w722, "error in"=w720) -> ("task out"=w712:refnum<k21>, "error out"=w713:errorcluster)  [unwired: 9 in]
            n511 = local write "write task"(w712) -> ()
          }
        }
      }
      frame #4 {
        n512 = while {
          tunnel: [w747] -> w727
          shift-right: [w748] -> w726
          shift-left: w725 -> [w751]
          i -> [w731]
          stop <- w749 stop-if-true
          # "debug: give stage time to move"
          # "This is the recording (looped for z-stacking).\nThe device is read out as fast as possible into a memory buffer,\nwhich is further averaged and transformed to the image."
          n513 = global read "xy_stack_global.vi" "Move to Y"() -> (w734:bool)
          n514 = Wait (ms)(milliseconds to wait=u32 500) -> (millisecond timer value=w728:u32)
          n515 = case shown="True" "Move to z" {
            tunnel: w751 -> [w757 w759]
            tunnel: [0.0 ("requested z-Position") w758] -> w736
            tunnel: [w757 w759] -> w739
            frame False {
            }
            frame True {
              # "This moves the stage to the current z-Position"
              n516 = local read "requested z-Position"() -> (w758:dbl)
              n517 = global write "MotorPosition.vi" "Request Z-Position"(w758) -> ()
            }
          }
          n518 = Increment(x=w731) -> (x+1=w730:i32)
          n519 = global read "xy_stack_global.vi" "Move to X"() -> (w735:bool)
          n520 = local write "Scan no."(w730) -> ()
          n521 = case shown="True" w735 {
            tunnel: [0.0 ("requested x-position") w755] -> w733
            tunnel: w728 -> [_ _]
            frame False {
            }
            frame True {
              n522 = global read "xy_stack_global.vi" "requested x-position"() -> (w755:dbl)
              n523 = global write "MotorPosition.vi" "Request X-Position"(w755) -> ()
            }
          }
          n524 = case shown="True" w734 {
            tunnel: [0.0 ("requested y-position") w753] -> w732
            frame False {
            }
            frame True {
              n525 = global read "xy_stack_global.vi" "requested y-position"() -> (w753:dbl)
              n526 = global write "MotorPosition.vi" "Request Y-Position"(w753) -> ()
            }
          }
          n527 = local read "Info File contents"() -> (w744:string)
          n528 = property on="z-Position" class="DigNum (strict)"("Value"=w736) -> ()  [unwired: 2 in, 2 out]
          n529 = Format Into String(format string="%.;Slide %d: x-pos: %f; y-pos: %f; z-pos: %f\n", initial string=w744, w730, w733, w732, w736) -> (resulting string=w743:string)  [unwired: 1 in, 1 out]
          n530 = local write "Info File contents"(w743) -> ()
          n531 = flat-sequence {
            tunnel: w739 -> [w769]
            tunnel: [w774] -> w750
            tunnel: [w773] -> w741
            tunnel: [w772] -> w740
            tunnel: [w770] -> w738
            tunnel: [w767] -> w737
            tunnel: w750 -> [w1359]
            tunnel: [w1360] -> w749
            tunnel: [w1356] -> w748
            tunnel: [w1339] -> w747
            tunnel: w746 -> [w1358]
            tunnel: w741 -> [w1357]
            tunnel: w740 -> [w1356]
            tunnel: w738 -> [w1355]
            tunnel: w737 -> [w1354]
            frame #0 {
              # "open the shutter\nunless a background is recorded"
              n532 = local read "Background"() -> (w761:bool)
              n533 = call-poly <vilib>:"DAQmx Create Virtual Channel.vi"("lines"=tag "Dev1/port2/line0", "error in"=w769) -> ("task out"=w765:refnum<k21>, "error out"=w762:errorcluster)  [unwired: 12 in]
              n534 = Not(x=w761) -> (.not. x?=w760:bool)
              n535 = call-poly <vilib>:"DAQmx Write.vi"("task/channels in"=w765, "data"=w760, "error in"=w762) -> ("task out"=w764:refnum<k21>, "error out"=w763:errorcluster)  [unwired: 10 in, 1 out]
              n536 = call <vilib>:"DAQmx Clear Task.vi"("task in"=w764, "error in"=w763) -> ("error out"=w768:errorcluster)  [unwired: 13 in]
              n537 = local read "Detector"() -> (w771:u16)
              n538 = case shown="0, Default" w771 {
                tunnel: [w820 w995 w1108 w1241] -> w774
                tunnel: [w819 i16[][] [] i16[][] [] i16[][] []] -> w773
                tunnel: [w797 w954 w1091 w1224] -> w772
                tunnel: w768 -> [w786 w994 w1107 w1240]
                tunnel: [u32[][][] [] w977 i16[][][] [] i16[][][] []] -> w770
                tunnel: [u32[][][] [] i16[][][] [] w1082 w1215] -> w767
                frame 0, Default {
                  # "Close the shutter"
                  # "Flyback"
                  n539 = local read "Number of pixels"() -> (w817:i32)
                  n540 = local read "scanning waveforms"() -> (w784:dbl[][])
                  n541 = local read "write task"() -> (w787:refnum<k21>)
                  n542 = call-poly <vilib>:"DAQmx Write.vi"("task/channels in"=w787, "auto start"=FALSE, "data"=w784, "error in"=w786) -> ("task out"=w790:refnum<k21>, "error out"=w789:errorcluster)  [unwired: 9 in, 1 out]
                  n543 = Initialize Array(0.0 ("element"), w817, w817) -> (w807:dbl[][])
                  n544 = Decrement(x=w817) -> (x-1=w809:i32)
                  n545 = Divide(x=w817, y=2) -> (x/y=w818:dbl)
                  n546 = Initialize Array(0.0 ("element"), w817, w818) -> (w808:dbl[][])
                  n547 = local read "read task"() -> (w794:refnum<k21>)
                  n548 = call <vilib>:"DAQmx Start Task.vi"("task/channels in"=w790, "error in"=w789) -> ("error out"=w785:errorcluster)  [unwired: 12 in, 1 out]
                  n549 = Obtain Queue(name (unnamed)="Buffer", element data type=i16 0) -> (queue out=w810:refnum<queue>)  [unwired: 3 in, 2 out]
                  n550 = Negate(x=w818) -> (-x=w811:dbl)
                  n551 = call <vilib>:"DAQmx Start Task.vi"("task/channels in"=w794, "error in"=w785) -> ("task out"=w792:refnum<k21>, "error out"=w793:errorcluster)  [unwired: 12 in]
                  n552 = while {
                    shift-right: [w867] -> _
                    shift-left: w809 -> [w871]
                    shift-right: [w860] -> _
                    shift-left: w809 -> [w870]
                    tunnel: w809 -> [w869]
                    shift-right: [w868] -> w820
                    shift-left: w807 -> [w872]
                    shift-right: [w866] -> w799
                    shift-left: w793 -> [w856]
                    tunnel: w811 -> [w865]
                    tunnel: w810 -> [w854]
                    shift-right: [w849] -> w819
                    shift-left: w808 -> [w850]
                    stop <- w862 stop-if-true
                    # "x-counter"
                    # "y-counter"
                    n553 = local read "Samples/Pixel"() -> (w858:u32)
                    n554 = Get Queue Status(queue=w854, error in (no error)=w856) -> (queue out=w853:refnum<queue>, error out=w857:errorcluster, # elements in queue=w855:i32)  [unwired: 1 in, 5 out]
                    n555 = Greater Or Equal?(x=w855, y=w858) -> (x >= y?=w873:bool)
                    n556 = case shown="True" w873 {
                      tunnel: w857 -> [w876 w887]
                      tunnel: w858 -> [_ w884]
                      tunnel: w872 -> [w877 w898]
                      tunnel: w871 -> [w879 w888]
                      tunnel: w870 -> [w878 w896]
                      tunnel: w869 -> [_ w895]
                      tunnel: [w877 w894] -> w868
                      tunnel: [w879 w893] -> w867
                      tunnel: [w878 w892] -> w860
                      tunnel: [w876 w886] -> w866
                      tunnel: w865 -> [_ w890]
                      tunnel: w853 -> [_ w885]
                      tunnel: [bool[] [FALSE] w882] -> w852
                      tunnel: w850 -> [w874 w881]
                      tunnel: [w874 w880] -> w849
                      frame False {
                      }
                      frame True {
                        n557 = for {
                          N: w884 -> [_]
                          tunnel: w885 -> [w901]
                          shift-right: [w902] -> w886
                          shift-left: w887 -> [w903]
                          tunnel: [w900] -> w883 mode=indexing
                          tunnel: [w899] -> w882 mode=indexing
                          n558 = Dequeue Element(queue=w901, error in (no error)=w903) -> (element=w900:i16, timed out?=w899:bool, error out=w902:errorcluster)  [unwired: 1 in, 1 out]
                        }
                        n559 = Greater Or Equal To 0?(x=w888) -> (x >= 0?=w889:bool)
                        n560 = Equal?(x=w890, y=w888) -> (x = y?=w891:bool)
                        n561 = case shown="True" w889 {
                          tunnel: w883 -> [w909 w918]
                          tunnel: w898 -> [w913 w924]
                          tunnel: w896 -> [w908 w921]
                          tunnel: [w913 w923] -> w894
                          tunnel: w888 -> [w906 w922]
                          tunnel: w881 -> [w910 w915]
                          tunnel: [w911 w915] -> w880
                          frame False {
                            n562 = Negate(x=w906) -> (-x=w907:i32)
                            n563 = call-poly <vilib>:"Mean.vi"("X"=w909) -> ("mean"=w912:dbl)  [unwired: 1 out]
                            n564 = Decrement(x=w907) -> (x-1=w905:i32)
                            n565 = Negate(x=w912) -> (-x=w904:dbl)
                            n566 = Replace Array Subset(array=w910, new element=w904, index (row)=w908, index (col)=w905) -> (w911:dbl[][])
                          }
                          frame True {
                            n567 = local read "Throw away"() -> (w917:bool)
                            n568 = case shown="True" w917 {
                              tunnel: w918 -> [w925 w928]
                              tunnel: [w925 w927] -> w919
                              frame False {
                              }
                              frame True {
                                n569 = local read "Thrown samples"() -> (w926:i16)
                                n570 = Array Subset(array=w928, index=w926) -> (w927:i16[])  [unwired: 1 in]
                              }
                            }
                            n571 = call-poly <vilib>:"Mean.vi"("X"=w919) -> ("mean"=w916:dbl)  [unwired: 1 out]
                            n572 = Negate(x=w916) -> (-x=w914:dbl)
                            n573 = To Word Integer(number=w914) -> (16bit integer=w920:i16)
                            n574 = Replace Array Subset(array=w924, new element=w920, index (row)=w921, index (col)=w922) -> (w923:dbl[][])
                          }
                        }
                        n575 = Decrement(x=w888) -> (x-1=w897:i32)
                        n576 = case shown="True" w891 {
                          tunnel: w896 -> [w930 w943]
                          tunnel: [w930 w942] -> w892
                          tunnel: w894 -> [_ w933]
                          tunnel: [w929 w944] -> w893
                          tunnel: w897 -> [w929 _]
                          tunnel: w895 -> [_ w944]
                          frame False {
                          }
                          frame True {
                            n577 = local read "Time per line [s]"() -> (w932:dbl)
                            n578 = Multiply(x=w932, y=w943) -> (x*y=w935:dbl)
                            n579 = Decrement(x=w943) -> (x-1=w942:i32)
                            n580 = Quotient & Remainder(x=w935, y=60.0) -> (x-y*floor(x/y)=w938:dbl, floor(x/y)=w940:dbl)
                            n581 = Divide(x=w938, y=100.0) -> (x/y=w939:dbl)
                            n582 = Add(x=w939, y=w940) -> (x+y=w936:dbl)
                            n583 = Number To Fractional String(number=w936, precision (6)=i16 2) -> (F-format string=w931:string)  [unwired: 2 in]
                            n584 = local write "Duration (m.s)"(w931) -> ()
                            "Image" <- w933
                          }
                        }
                      }
                    }
                    n585 = Or Array Elements(Boolean array=w852) -> (logical OR=w851:bool)
                    n586 = local read "Scan"() -> (w859:bool)
                    n587 = Not(x=w859) -> (.not. x?=w861:bool)
                    n588 = Unbundle By Name(w866) -> ("status"=w864:bool)
                    n589 = Less Than 0?(x=w860) -> (x < 0?=w863:bool)
                    n590 = Compound Arithmetic op=OR(w864, w863, w861, w851) -> (w862:bool)
                  }
                  n591 = while {
                    shift-right: [w830] -> w798
                    shift-left: w793 -> [w843]
                    tunnel: w810 -> [w829]
                    tunnel: [w822] -> w795
                    tunnel: w792 -> [w821]
                    stop <- w841 stop-if-true
                    w842 = -1.0 ("timeout")
                    n592 = call-poly <vilib>:"DAQmx Read.vi"("task/channels in"=w821, "number of samples per channel"=w842, "timeout"=w842, "error in"=w843) -> ("task out"=w838:refnum<k21>, "data"=w825:i16[], "error out"=w828:errorcluster)  [unwired: 9 in]
                    n593 = Array Size(array=w825) -> (size(s)=w826:i32)
                    n594 = for {
                      N: w826 -> [_]
                      tunnel: w829 -> [w848]
                      shift-right: [w846] -> w827
                      shift-left: w828 -> [w847]
                      tunnel: w825 -> [w845] mode=indexing
                      tunnel: [w844] -> w824 mode=indexing
                      n595 = Enqueue Element(queue=w848, element=w845, error in (no error)=w847) -> (timed out?=w844:bool, error out=w846:errorcluster)  [unwired: 1 in, 1 out]
                    }
                    n596 = Or Array Elements(Boolean array=w824) -> (logical OR=w823:bool)
                    n597 = call <vilib>:"DAQmx Is Task Done.vi"("task/channels in"=w838, "error in"=w827) -> ("task out"=w833:refnum<k21>, "task done?"=w835:bool, "error out"=w832:errorcluster)  [unwired: 11 in]
                    n598 = property class="DAQmx Read"(reference=w833, error in=w832) -> (reference out=w822:refnum<k21>, error out=w830:errorcluster, "AvailSampPerChan"=w837:u32)
                    n599 = Equal To 0?(x=w837) -> (x = 0?=w836:bool)
                    n600 = local read "Scan"() -> (w831:bool)
                    n601 = And(x=w836, y=w835) -> (x .and. y?=w834:bool)
                    n602 = Unbundle By Name(w830) -> ("status"=w840:bool)
                    n603 = Not(x=w831) -> (.not. x?=w839:bool)
                    n604 = Compound Arithmetic op=OR(w840, w839, w834, w823) -> (w841:bool)
                  }
                  n605 = call <vilib>:"DAQmx Stop Task.vi"("task/channels in"=w795, "error in"=w798) -> ("error out"=w777:errorcluster)  [unwired: 12 in, 1 out]
                  n606 = local read "write task"() -> (w806:refnum<k21>)
                  n607 = call <vilib>:"DAQmx Stop Task.vi"("task/channels in"=w806, "error in"=w799) -> ("error out"=w796:errorcluster)  [unwired: 12 in, 1 out]
                  n608 = call-poly <vilib>:"DAQmx Create Virtual Channel.vi"("lines"=tag "Dev1/port2/line0", "error in"=w777) -> ("task out"=w779:refnum<k21>, "error out"=w780:errorcluster)  [unwired: 12 in]
                  n609 = call-poly <vilib>:"DAQmx Write.vi"("task/channels in"=w779, "data"=FALSE, "error in"=w780) -> ("task out"=w782:refnum<k21>, "error out"=w783:errorcluster)  [unwired: 10 in, 1 out]
                  n610 = call <vilib>:"DAQmx Clear Task.vi"("task in"=w782, "error in"=w783) -> ("error out"=w776:errorcluster)  [unwired: 13 in]
                  n611 = Merge Errors(w796, w777, w776) -> (w800:errorcluster)
                  n612 = Obtain Queue(name (unnamed)="Buffer", element data type=i16 0, error in (no error)=w800) -> (queue out=w803:refnum<queue>, error out=w801:errorcluster)  [unwired: 2 in, 1 out]
                  n613 = Release Queue(queue=w803, force destroy? (F)=TRUE, error in (no error)=w801) -> (error out=w797:errorcluster)  [unwired: 2 out]
                }
                frame 1 {
                  # "Close the shutter"
                  # "Flyback"
                  n614 = local read "Number of pixels"() -> (w980:i32)
                  n615 = local read "scanning waveforms"() -> (w950:dbl[][])
                  n616 = call "Maya2000 - Open all.vi"() -> ("error out"=w991:errorcluster, ".NET Refnum out"=w993:refnum<k24>, "Maya2000 Basic \n[UV2400,UV600]"=w992:T7[])  [unwired: 9 in]
                  n617 = call "Maya2000 - set N coadd and integr time.vi"("Intgration time\n[us]"="Intgration time [us]", "error in (no error)"=w991, "Maya2000 basic values"=w992, ".NET Refnum in"=w993) -> ("error out"=w987:errorcluster, "This instruments index"=w984:i32, ".NET Refnum out"=w986:refnum<k24>)  [unwired: 4 in, 1 out]
                  n618 = Initialize Array(0.0 ("element"), w980, w980) -> (w996:dbl[][])
                  n619 = Decrement(x=w980) -> (x-1=w982:i32)
                  n620 = invoke class="NETWrapper" method="getWavelengths"(reference=w986, error in=w987, "spectrometerIndex"=w984) -> (reference out=w985:refnum<k24>, error out=w983:errorcluster, "getWavelengths"=w967:dbl[])  [unwired: 1 in, 1 out]
                  n621 = Array Size(array=w967) -> (size(s)=w978:i32)
                  n622 = Initialize Array(u32 0 ("element"), w980, w980, w978) -> (w979:u32[][][])
                  n623 = Divide(x=w980, y=2) -> (x/y=w1000:dbl)
                  n624 = Negate(x=w1000) -> (-x=w997:dbl)
                  n625 = Subtract(x=w967, y="Wavelength min") -> (x-y=w972:dbl[])
                  n626 = Subtract(x=w967, y="Wavelength max") -> (x-y=w969:dbl[])
                  n627 = Index Array(array=w950, index (row)=0) -> (element=w947:dbl[])  [unwired: 1 in]
                  n628 = Index Array(array=w950, index (row)=1) -> (element=w946:dbl[])  [unwired: 1 in]
                  n629 = Absolute Value(x=w972) -> (abs(x)=w971:dbl[])
                  n630 = Absolute Value(x=w969) -> (abs(x)=w968:dbl[])
                  n631 = Array Max & Min(array=w971) -> (min index (indices)=w966:i32)  [unwired: 3 out]
                  n632 = Array Max & Min(array=w968) -> (min index (indices)=w965:i32)  [unwired: 3 out]
                  n633 = Decimate 1D Array(w947) -> (w975:dbl[])  [unwired: 1 out]
                  n634 = Decimate 1D Array(w946) -> (w974:dbl[])  [unwired: 1 out]
                  n635 = Subtract(x=w965, y=w966) -> (x-y=w964:i32)
                  n636 = for {
                    tunnel: w997 -> [w1036]
                    shift-right: [w1019] -> w952
                    shift-left: w994 -> [w1011]
                    tunnel: w985 -> [w1018]
                    tunnel: w984 -> [w1017]
                    tunnel: [w1016] -> w988
                    tunnel: w983 -> [_]
                    shift-right: [w1026] -> w995
                    shift-left: w996 -> [w1033]
                    shift-right: [w1030] -> _
                    shift-left: w982 -> [w1034]
                    tunnel: w982 -> [w1027]
                    shift-right: [w1028] -> _
                    shift-left: w982 -> [w1029]
                    shift-right: [w1020] -> w977
                    shift-left: w979 -> [w1021]
                    tunnel: w975 -> [w1013] mode=indexing
                    tunnel: w974 -> [w1012] mode=indexing
                    tunnel: w966 -> [w1015]
                    tunnel: w964 -> [w1014]
                    stop <- w1023 stop-if-true
                    # "x-counter"
                    # "y-counter"
                    n637 = Equal?(x=w1036, y=w1034) -> (x = y?=w1032:bool)
                    n638 = Decrement(x=w1034) -> (x-1=w1031:i32)
                    n639 = Greater Or Equal To 0?(x=w1034) -> (x >= 0?=w1035:bool)
                    n640 = local read "write task"() -> (w1009:refnum<k21>)
                    n641 = Build Array(w1013, w1012) -> (w1008:dbl[])
                    n642 = call-poly <vilib>:"DAQmx Write.vi"("task/channels in"=w1009, "auto start"=TRUE, "data"=w1008, "error in"=w1011) -> ("number of samples written per channel"=w1006:u32, "error out"=w1010:errorcluster)  [unwired: 9 in, 1 out]
                    n643 = local read "Intgration time [us]"() -> (w1002:u32)
                    n644 = Divide(x=w1002, y=u32 1000) -> (x/y=w1003:dbl)
                    n645 = Multiply(x=w1003, y=w1006) -> (x*y=w1004:dbl)
                    n646 = Wait (ms)(milliseconds to wait=w1004) -> (millisecond timer value=w1005:u32)
                    n647 = case shown="True" w1035 {
                      tunnel: w1034 -> [_ w1068]
                      tunnel: w1029 -> [_ w1069]
                      tunnel: w1033 -> [w1056 w1072]
                      tunnel: [w1056 w1071] -> w1026
                      tunnel: w1021 -> [w1055 w1070]
                      tunnel: [w1055 w1067] -> w1020
                      tunnel: w1010 -> [w1053 w1065]
                      tunnel: [w1053 w1064] -> w1019
                      tunnel: w1018 -> [w1054 w1063]
                      tunnel: w1017 -> [_ w1062]
                      tunnel: [w1054 w1061] -> w1016
                      tunnel: w1015 -> [_ w1058]
                      tunnel: w1014 -> [_ w1057]
                      tunnel: w1005 -> [_ _]
                      frame False {
                      }
                      frame True {
                        n648 = invoke class="NETWrapper" method="getSpectrum"(reference=w1063, error in=w1065, "spectrometerIndex"=w1062) -> (reference out=w1061:refnum<k24>, error out=w1064:errorcluster, "getSpectrum"=w1060:dbl[])  [unwired: 1 in, 1 out]
                        n649 = Replace Array Subset(array=w1070, new element=w1060, index (dim 0)=w1069, index (dim 1)=w1068) -> (w1067:u32[][][])  [unwired: 1 in]
                        n650 = Array Subset(array=w1060, index=w1058, length=w1057) -> (w1059:dbl[])
                        n651 = call-poly <vilib>:"Mean.vi"("X"=w1059) -> ("mean"=w1066:dbl)  [unwired: 1 out]
                        n652 = Replace Array Subset(array=w1072, new element=w1066, index (row)=w1069, index (col)=w1068) -> (w1071:dbl[][])
                      }
                    }
                    n653 = case shown="True" w1032 {
                      tunnel: w1031 -> [w1038 _]
                      tunnel: [w1038 w1051] -> w1030
                      tunnel: w1029 -> [w1037 w1042]
                      tunnel: [w1037 w1052] -> w1028
                      tunnel: w1027 -> [_ w1051]
                      tunnel: w1026 -> [_ w1039]
                      frame False {
                      }
                      frame True {
                        n654 = local read "Time per line [s]"() -> (w1040:dbl)
                        n655 = Decrement(x=w1042) -> (x-1=w1052:i32)
                        n656 = Multiply(x=w1040, y=w1042) -> (x*y=w1044:dbl)
                        n657 = Quotient & Remainder(x=w1044, y=60.0) -> (x-y*floor(x/y)=w1047:dbl, floor(x/y)=w1049:dbl)
                        n658 = Divide(x=w1047, y=100.0) -> (x/y=w1048:dbl)
                        n659 = Add(x=w1048, y=w1049) -> (x+y=w1045:dbl)
                        n660 = Number To Fractional String(number=w1045, precision (6)=i16 2) -> (F-format string=w1041:string)  [unwired: 2 in]
                        n661 = local write "Duration (m.s)"(w1041) -> ()
                        n662 = local write "Image"(w1039) -> ()
                      }
                    }
                    n663 = local read "Scan"() -> (w1025:bool)
                    n664 = Unbundle By Name(w1019) -> ("status"=w1022:bool)
                    n665 = Not(x=w1025) -> (.not. x?=w1024:bool)
                    n666 = Or(x=w1022, y=w1024) -> (x .or. y?=w1023:bool)
                  }
                  n667 = local read "write task"() -> (w953:refnum<k21>)
                  n668 = call "Maya2000 - Close all.vi"("error in (no error)"=w952, "Maya reference in"=w988) -> ("error out"=w990:errorcluster, ".NET Refnum out"=w989:refnum<k24>)  [unwired: 8 in]
                  n669 = call <vilib>:"DAQmx Stop Task.vi"("task/channels in"=w953, "error in"=w952) -> ("error out"=w951:errorcluster)  [unwired: 12 in, 1 out]
                  n670 = call-poly <vilib>:"DAQmx Create Virtual Channel.vi"("lines"=tag "Dev1/port2/line0", "error in"=w952) -> ("task out"=w958:refnum<k21>, "error out"=w959:errorcluster)  [unwired: 12 in]
                  n671 = Close Reference(reference=w989, error in (no error)=w990) -> (error out=w955:errorcluster)
                  n672 = call-poly <vilib>:"DAQmx Write.vi"("task/channels in"=w958, "data"=FALSE, "error in"=w959) -> ("task out"=w961:refnum<k21>, "error out"=w962:errorcluster)  [unwired: 10 in, 1 out]
                  n673 = call <vilib>:"DAQmx Clear Task.vi"("task in"=w961, "error in"=w962) -> ("error out"=w956:errorcluster)  [unwired: 13 in]
                  n674 = Merge Errors(w955, w956, w951) -> (w954:errorcluster)
                }
                frame 2 {
                  # "maybe not constant\ntake value from somewhere"
                  # "Close the shutter"
                  # "Flyback"
                  n675 = local read "scanning waveforms"() -> (w1088:dbl[][])
                  n676 = local read "Number of pixels"() -> (w1104:i32)
                  n677 = Initialize Array(0.0 ("element"), w1104, w1104) -> (w1109:dbl[][])
                  n678 = Initialize Array(0.0 ("element"), w1104, w1104, 1024 ("dimension size")) -> (w1103:dbl[][][])
                  n679 = Decrement(x=w1104) -> (x-1=w1106:i32)
                  n680 = Divide(x=w1104, y=2) -> (x/y=w1113:dbl)
                  n681 = call "init.vi"() -> ("Image"=w1076:T8, "IMAQ Session Out"=w1079:refnum<k11>, "Buffer Handle"=w1078:T8, "Image Type"=w1075:u32)  [unwired: 7 in, 1 out]
                  n682 = local read "OCM Settings"() -> (w1073:T1)
                  n683 = Negate(x=w1113) -> (-x=w1110:dbl)
                  n684 = Index Array(array=w1088, index (row)=0) -> (element=w1085:dbl[])  [unwired: 1 in]
                  n685 = Index Array(array=w1088, index (row)=1) -> (element=w1084:dbl[])  [unwired: 1 in]
                  n686 = Equal To 0?(x=w1075) -> (x = 0?=w1074:bool)
                  n687 = Decimate 1D Array(w1085) -> (w1101:dbl[])  [unwired: 1 out]
                  n688 = Decimate 1D Array(w1084) -> (w1100:dbl[])  [unwired: 1 out]
                  n689 = for {
                    tunnel: w1110 -> [w1151]
                    shift-right: [w1120] -> w1081
                    shift-left: w1107 -> [w1131]
                    tunnel: [w1134] -> w1080
                    shift-right: [w1141] -> w1108
                    shift-left: w1109 -> [w1148]
                    shift-right: [w1145] -> _
                    shift-left: w1106 -> [w1149]
                    tunnel: w1106 -> [w1142]
                    shift-right: [w1143] -> _
                    shift-left: w1106 -> [w1144]
                    shift-right: [w1135] -> w1082
                    shift-left: w1103 -> [w1136]
                    tunnel: w1101 -> [w1133] mode=indexing
                    tunnel: w1100 -> [w1132] mode=indexing
                    tunnel: w1079 -> [w1119]
                    tunnel: w1076 -> [w1118]
                    tunnel: w1074 -> [w1117]
                    tunnel: w1073 -> [w1116]
                    stop <- w1138 stop-if-true
                    # "should become right\nas soon as trigger"
                    # "reading the wrong \nbuffer no?"
                    # "3D OCM Array"
                    # "2D Image"
                    # "x-counter"
                    # "y-counter"
                    n690 = Unbundle By Name(w1116) -> ("FFT AVG Size"=w1115:dbl, "Pixels FFT"=w1114:i32)
                    n691 = local read "write task"() -> (w1129:refnum<k21>)
                    n692 = Equal?(x=w1151, y=w1149) -> (x = y?=w1147:bool)
                    n693 = Decrement(x=w1149) -> (x-1=w1146:i32)
                    n694 = Greater Or Equal To 0?(x=w1149) -> (x >= 0?=w1150:bool)
                    n695 = Build Array(w1133, w1132) -> (w1128:dbl[])
                    n696 = call-poly <vilib>:"DAQmx Write.vi"("task/channels in"=w1129, "auto start"=TRUE, "data"=w1128, "error in"=w1131) -> ("number of samples written per channel"=w1126:u32, "error out"=w1130:errorcluster)  [unwired: 9 in, 1 out]
                    n697 = local read "Intgration time [us]"() -> (w1122:u32)
                    n698 = Divide(x=w1122, y=u32 10000) -> (x/y=w1123:dbl)
                    n699 = Multiply(x=w1123, y=w1126) -> (x*y=w1124:dbl)
                    n700 = Wait (ms)(milliseconds to wait=w1124) -> (millisecond timer value=w1125:u32)
                    n701 = case shown="True" w1150 {
                      tunnel: w1149 -> [_ w1186]
                      tunnel: w1144 -> [_ w1187]
                      tunnel: w1148 -> [w1163 w1190]
                      tunnel: [w1163 w1189] -> w1141
                      tunnel: w1136 -> [w1162 w1188]
                      tunnel: [w1162 w1185] -> w1135
                      tunnel: w1130 -> [w1161 w1181]
                      tunnel: [w1161 w1182] -> w1120
                      tunnel: [w1160 w1179] -> w1134
                      tunnel: w1125 -> [_ _]
                      tunnel: w1119 -> [w1160 w1180]
                      tunnel: w1118 -> [_ w1176]
                      tunnel: w1117 -> [_ w1175]
                      tunnel: w1116 -> [_ w1170]
                      tunnel: w1115 -> [_ w1166]
                      tunnel: w1114 -> [_ w1169]
                      tunnel: w1114 -> [_ w1167]
                      frame False {
                      }
                      frame True {
                        n702 = Initialize Array(0.0, w1166, w1167) -> (w1165:dbl[][])
                        n703 = for {
                          N: w1166 -> [_]
                          tunnel: w1176 -> [w1197]
                          tunnel: w1175 -> [w1196]
                          tunnel: [w1195] -> w1164
                          tunnel: w1170 -> [w1194]
                          shift-right: [w1202] -> w1182
                          shift-left: w1181 -> [w1201]
                          shift-right: [w1199] -> w1179
                          shift-left: w1180 -> [w1200]
                          shift-right: [w1191] -> _
                          shift-left: w1165 -> [w1192]
                          i -> [w1193]
                          # "Multiple OCM meas. to AVG"
                          n704 = call <vilib>:"IMAQ Copy Acquired Buffer.vi"("IMAQ Session In"=w1200, "Image In"=w1197, "Buffer Number"=w1193, "error in (no error)"=w1201) -> ("IMAQ Session Out"=w1199:refnum<k11>, "Image Out"=w1204:T8, "error out"=w1203:errorcluster)  [unwired: 7 in, 2 out]
                          n705 = call "IMAQ ImageToArray"("error in (no error)"=w1203, "Image"=w1204) -> ("Image Pixels (U16)"=w1205:u16[][], "error out"=w1202:errorcluster, "Image Pixels (U8)"=w1206:u8[][])  [unwired: 2 in, 2 out]
                          n706 = Select(t=w1206, s=w1196, f=w1205) -> (s? t:f=w1198:u16[][])
                          n707 = call "postprocess.vi"("FFT AVG Buffer IN"=w1192, "OCM Settings"=w1194, "Image Pixels"=w1198) -> ("AVG Buffer OUT"=w1191:dbl[][], "FFT Processed"=w1195:dbl[])  [unwired: 4 in, 3 out]
                        }
                        n708 = Replace Array Subset(array=w1188, new element=w1164, index (dim 0)=w1187, index (dim 1)=w1186) -> (w1185:dbl[][][])  [unwired: 1 in]
                        n709 = Decrement(x=w1169) -> (x-1=w1173:i32)
                        n710 = call-poly <vilib>:"Ramp Pattern.vi"("start"=0.0, "end"=w1173, "samples"=w1169) -> ("Ramp Pattern"=w1171:dbl[])  [unwired: 7 in, 1 out]
                        n711 = Array Subset(array=w1164, index="FFT index", length="length") -> (w1183:dbl[])
                        n712 = call-poly <vilib>:"Mean.vi"("X"=w1183) -> ("mean"=w1184:dbl)  [unwired: 1 out]
                        n713 = Replace Array Subset(array=w1190, new element=w1184, index (row)=w1187, index (col)=w1186) -> (w1189:dbl[][])
                        n714 = Bundle("Ramp Pattern"=w1171, "FFT Processed"=w1164) -> (→"Processed FFT":T9)  [unwired: 1 in]
                      }
                    }
                    n715 = case shown="True" w1147 {
                      tunnel: w1146 -> [w1153 _]
                      tunnel: [w1153 w1158] -> w1145
                      tunnel: w1144 -> [w1152 w1154]
                      tunnel: [w1152 w1159] -> w1143
                      tunnel: w1142 -> [_ w1158]
                      tunnel: w1141 -> [_ w1157]
                      frame False {
                      }
                      frame True {
                        n716 = local read "Time per line [s]"() -> (w1155:dbl)
                        n717 = call "scan_duration.vi"("x-counter"=w1154, "Time per Line"=w1155) -> ("Duration (m.s)"=w1156:string)
                        n718 = Decrement(x=w1154) -> (x-1=w1159:i32)
                        n719 = local write "Duration (m.s)"(w1156) -> ()
                        n720 = local write "Image"(w1157) -> ()
                      }
                    }
                    n721 = Unbundle By Name(w1120) -> ("status"=w1137:bool)
                    n722 = local read "Scan"() -> (w1140:bool)
                    n723 = Not(x=w1140) -> (.not. x?=w1139:bool)
                    n724 = Or(x=w1137, y=w1139) -> (x .or. y?=w1138:bool)
                  }
                  n725 = local read "write task"() -> (w1090:refnum<k21>)
                  n726 = call "BASLER_stop.vi"("error in (no error)"=w1081, "Image"=w1076, "Buffer Handle"=w1078, "IMAQ Session"=w1080) -> ("error out"=w1092:errorcluster)  [unwired: 7 in]
                  n727 = call <vilib>:"DAQmx Stop Task.vi"("task/channels in"=w1090, "error in"=w1081) -> ("error out"=w1089:errorcluster)  [unwired: 12 in, 1 out]
                  n728 = call-poly <vilib>:"DAQmx Create Virtual Channel.vi"("lines"=tag "Dev1/port2/line0", "error in"=w1081) -> ("task out"=w1095:refnum<k21>, "error out"=w1096:errorcluster)  [unwired: 12 in]
                  n729 = call-poly <vilib>:"DAQmx Write.vi"("task/channels in"=w1095, "data"=FALSE, "error in"=w1096) -> ("task out"=w1098:refnum<k21>, "error out"=w1099:errorcluster)  [unwired: 10 in, 1 out]
                  n730 = call <vilib>:"DAQmx Clear Task.vi"("task in"=w1098, "error in"=w1099) -> ("error out"=w1093:errorcluster)  [unwired: 13 in]
                  n731 = Merge Errors(w1092, w1093, w1089) -> (w1091:errorcluster)
                }
                frame 3 {
                  # "maybe not constant\ntake value from somewhere"
                  # "Close the shutter"
                  # "Flyback"
                  n732 = local read "scanning waveforms"() -> (w1221:dbl[][])
                  n733 = local read "Number of pixels"() -> (w1237:i32)
                  n734 = Initialize Array(0.0 ("element"), w1237, w1237) -> (w1242:dbl[][])
                  n735 = Initialize Array(0.0 ("element"), w1237, w1237, 1024 ("dimension size")) -> (w1236:dbl[][][])
                  n736 = Decrement(x=w1237) -> (x-1=w1239:i32)
                  n737 = Divide(x=w1237, y=2) -> (x/y=w1246:dbl)
                  n738 = call "init.vi"() -> ("Image"=w1209:T8, "IMAQ Session Out"=w1212:refnum<k11>, "Buffer Handle"=w1211:T8, "Image Type"=w1208:u32)  [unwired: 7 in, 1 out]
                  n739 = Negate(x=w1246) -> (-x=w1243:dbl)
                  n740 = Index Array(array=w1221, index (row)=0) -> (element=w1218:dbl[])  [unwired: 1 in]
                  n741 = Index Array(array=w1221, index (row)=1) -> (element=w1217:dbl[])  [unwired: 1 in]
                  n742 = Equal To 0?(x=w1208) -> (x = 0?=w1207:bool)
                  n743 = Decimate 1D Array(w1218) -> (w1234:dbl[])  [unwired: 1 out]
                  n744 = Decimate 1D Array(w1217) -> (w1233:dbl[])  [unwired: 1 out]
                  n745 = for {
                    tunnel: w1243 -> [w1281]
                    shift-right: [w1250] -> w1214
                    shift-left: w1240 -> [w1261]
                    tunnel: [w1264] -> w1213
                    shift-right: [w1271] -> w1241
                    shift-left: w1242 -> [w1278]
                    shift-right: [w1275] -> _
                    shift-left: w1239 -> [w1279]
                    tunnel: w1239 -> [w1272]
                    shift-right: [w1273] -> _
                    shift-left: w1239 -> [w1274]
                    shift-right: [w1265] -> w1215
                    shift-left: w1236 -> [w1266]
                    tunnel: w1234 -> [w1263] mode=indexing
                    tunnel: w1233 -> [w1262] mode=indexing
                    tunnel: w1212 -> [w1249]
                    tunnel: w1209 -> [w1248]
                    tunnel: w1207 -> [w1247]
                    stop <- w1268 stop-if-true
                    # "should become right\nas soon as trigger"
                    # "reading the wrong \nbuffer no?"
                    # "3D OCM Array"
                    # "2D Image"
                    # "x-counter"
                    # "y-counter"
                    n746 = local read "write task"() -> (w1259:refnum<k21>)
                    n747 = Equal?(x=w1281, y=w1279) -> (x = y?=w1277:bool)
                    n748 = Decrement(x=w1279) -> (x-1=w1276:i32)
                    n749 = Greater Or Equal To 0?(x=w1279) -> (x >= 0?=w1280:bool)
                    n750 = Build Array(w1263, w1262) -> (w1258:dbl[])
                    n751 = call-poly <vilib>:"DAQmx Write.vi"("task/channels in"=w1259, "auto start"=TRUE, "data"=w1258, "error in"=w1261) -> ("number of samples written per channel"=w1256:u32, "error out"=w1260:errorcluster)  [unwired: 9 in, 1 out]
                    n752 = local read "Intgration time [us]"() -> (w1252:u32)
                    n753 = Divide(x=w1252, y=u32 10000) -> (x/y=w1253:dbl)
                    n754 = Multiply(x=w1253, y=w1256) -> (x*y=w1254:dbl)
                    n755 = Wait (ms)(milliseconds to wait=w1254) -> (millisecond timer value=w1255:u32)
                    n756 = case shown="True" w1280 {
                      tunnel: w1279 -> [_ w1309]
                      tunnel: w1274 -> [_ w1310]
                      tunnel: w1278 -> [w1293 w1313]
                      tunnel: [w1293 w1312] -> w1271
                      tunnel: w1266 -> [w1292 w1311]
                      tunnel: [w1292 w1308] -> w1265
                      tunnel: w1260 -> [w1291 w1305]
                      tunnel: [w1291 w1306] -> w1250
                      tunnel: [w1290 w1303] -> w1264
                      tunnel: w1255 -> [_ _]
                      tunnel: w1249 -> [w1290 w1304]
                      tunnel: w1248 -> [_ w1302]
                      tunnel: w1247 -> [_ w1301]
                      frame False {
                      }
                      frame True {
                        # "Multiple OCM meas. to AVG"
                        n757 = call <vilib>:"IMAQ Copy Acquired Buffer.vi"("IMAQ Session In"=w1304, "Image In"=w1302, "error in (no error)"=w1305) -> ("IMAQ Session Out"=w1303:refnum<k11>, "Image Out"=w1298:T8, "error out"=w1297:errorcluster)  [unwired: 8 in, 2 out]
                        n758 = call "IMAQ ImageToArray"("error in (no error)"=w1297, "Image"=w1298) -> ("Image Pixels (U16)"=w1299:u16[][], "error out"=w1306:errorcluster, "Image Pixels (U8)"=w1300:u8[][])  [unwired: 2 in, 2 out]
                        n759 = Select(t=w1300, s=w1301, f=w1299) -> (s? t:f=w1295:u16[][])
                        n760 = Transpose 2D Array(2D array=w1295) -> (transposed array=w1296:u16[][])
                        n761 = for {
                          tunnel: w1296 -> [w1315] mode=indexing
                          tunnel: [w1314] -> w1294 mode=indexing
                          n762 = call-poly <vilib>:"Mean.vi"("X"=w1315) -> ("mean"=w1314:dbl)  [unwired: 1 out]
                        }
                        n763 = Replace Array Subset(array=w1311, new element=w1294, index (dim 0)=w1310, index (dim 1)=w1309) -> (w1308:dbl[][][])  [unwired: 1 in]
                        n764 = call-poly <vilib>:"Mean.vi"("X"=w1294) -> ("mean"=w1307:dbl)  [unwired: 1 out]
                        n765 = Replace Array Subset(array=w1313, new element=w1307, index (row)=w1310, index (col)=w1309) -> (w1312:dbl[][])
                      }
                    }
                    n766 = case shown="True" w1277 {
                      tunnel: w1276 -> [w1283 _]
                      tunnel: [w1283 w1288] -> w1275
                      tunnel: w1274 -> [w1282 w1284]
                      tunnel: [w1282 w1289] -> w1273
                      tunnel: w1272 -> [_ w1288]
                      tunnel: w1271 -> [_ w1287]
                      frame False {
                      }
                      frame True {
                        n767 = local read "Time per line [s]"() -> (w1285:dbl)
                        n768 = call "scan_duration.vi"("x-counter"=w1284, "Time per Line"=w1285) -> ("Duration (m.s)"=w1286:string)
                        n769 = Decrement(x=w1284) -> (x-1=w1289:i32)
                        n770 = local write "Duration (m.s)"(w1286) -> ()
                        n771 = local write "Image"(w1287) -> ()
                      }
                    }
                    n772 = Unbundle By Name(w1250) -> ("status"=w1267:bool)
                    n773 = local read "Scan"() -> (w1270:bool)
                    n774 = Not(x=w1270) -> (.not. x?=w1269:bool)
                    n775 = Or(x=w1267, y=w1269) -> (x .or. y?=w1268:bool)
                  }
                  n776 = local read "write task"() -> (w1223:refnum<k21>)
                  n777 = call "BASLER_stop.vi"("error in (no error)"=w1214, "Image"=w1209, "Buffer Handle"=w1211, "IMAQ Session"=w1213) -> ("error out"=w1225:errorcluster)  [unwired: 7 in]
                  n778 = call <vilib>:"DAQmx Stop Task.vi"("task/channels in"=w1223, "error in"=w1214) -> ("error out"=w1222:errorcluster)  [unwired: 12 in, 1 out]
                  n779 = call-poly <vilib>:"DAQmx Create Virtual Channel.vi"("lines"=tag "Dev1/port2/line0", "error in"=w1214) -> ("task out"=w1228:refnum<k21>, "error out"=w1229:errorcluster)  [unwired: 12 in]
                  n780 = call-poly <vilib>:"DAQmx Write.vi"("task/channels in"=w1228, "data"=FALSE, "error in"=w1229) -> ("task out"=w1231:refnum<k21>, "error out"=w1232:errorcluster)  [unwired: 10 in, 1 out]
                  n781 = call <vilib>:"DAQmx Clear Task.vi"("task in"=w1231, "error in"=w1232) -> ("error out"=w1226:errorcluster)  [unwired: 13 in]
                  n782 = Merge Errors(w1225, w1226, w1222) -> (w1224:errorcluster)
                }
              }
            }
            frame #1 {
              w1316 = FALSE
              # "stop if yx done no z"
              n783 = local read "xy-Stacking"() -> (w1336:bool)
              n784 = global read "xy_stack_global.vi" "# steps X"() -> (w1347:u16)
              n785 = global read "xy_stack_global.vi" "# steps Y"() -> (w1352:u16)
              n786 = local read "Scan no."() -> (w1321:i32)
              n787 = local read "xy-Stacking"() -> (w1349:bool)
              n788 = global read "xy_stack_global.vi" "# steps X"() -> (w1335:u16)
              n789 = local read "Scan no."() -> (w1318:i32)
              n790 = Increment(x=w1352) -> (x+1=w1351:u16)
              n791 = Increment(x=w1335) -> (x+1=w1350:u16)
              n792 = Multiply(x=w1350, y=w1351) -> (x*y=w1319:u16)
              n793 = Increment(x=w1347) -> (x+1=w1320:u16)
              n794 = Not(x=w1336) -> (.not. x?=w1353:bool)
              n795 = Quotient & Remainder(x=w1318, y=w1319) -> (x-y*floor(x/y)=w1333:i32)  [unwired: 1 out]
              n796 = Quotient & Remainder(x=w1321, y=w1320) -> (x-y*floor(x/y)=w1346:i32, floor(x/y)=→"floor(x/y)":i32)
              n797 = Equal?(x=w1333, y=0) -> (x = y?=w1332:bool)
              n798 = local read "z-Stacking"() -> (w1340:bool)
              n799 = Equal?(x=w1346, y=0) -> (x = y?=w1344:bool)
              n800 = Not(x=w1344) -> (.not. x?=w1348:bool)
              n801 = Or(x=w1332, y=w1353) -> (x .or. y?=w1325:bool)
              n802 = local read "Save"() -> (w1363:bool)
              n803 = local write "Background"(w1316) -> ()
              n804 = And(x=w1349, y=w1348) -> (x .and. y?=w1338:bool)
              n805 = Compound Arithmetic op=AND(w1340, w1325) -> (w1341:bool)
              n806 = property on="Laser Blocking" class="Str"("Visible"=w1316) -> ()  [unwired: 2 in, 2 out]
              n807 = case shown="False" w1341 {
                tunnel: [w1368 w1377] -> w1342
                tunnel: w1338 -> [w1367 _]
                tunnel: [w1366 w1379] -> w1337
                tunnel: [w1365 w1378] -> w1326
                frame False {
                  n808 = case shown="False" w1367 {
                    tunnel: [w1370 w1374] -> w1366
                    tunnel: [w1369 w1373] -> w1365
                    frame False {
                      n809 = global read "xy_stack_global.vi" "requested y-position"() -> (w1372:dbl)
                      n810 = global read "xy_stack_global.vi" "X-Minimum"() -> (w1370:dbl)
                      n811 = global read "xy_stack_global.vi" "Step size Y"() -> (w1371:dbl)
                      n812 = Add(x=w1372, y=w1371) -> (x+y=w1369:dbl)
                    }
                    frame True {
                      # "increment x every step OR \nincrement y (and reset x)"
                      n813 = global read "xy_stack_global.vi" "requested x-position"() -> (w1376:dbl)
                      n814 = global read "xy_stack_global.vi" "requested y-position"() -> (w1373:dbl)
                      n815 = global read "xy_stack_global.vi" "Step size X"() -> (w1375:dbl)
                      n816 = Add(x=w1375, y=w1376) -> (x+y=w1374:dbl)
                    }
                  }
                  n817 = local read "requested z-Position"() -> (w1368:dbl)
                }
                frame True {
                  # "increment z at #xsteps*#ysteps\nreset X and Y"
                  n818 = local read "requested z-Position"() -> (w1383:dbl)
                  n819 = local read "# steps"() -> (w1381:u16)
                  n820 = local read "Step size"() -> (w1382:dbl)
                  n821 = global read "xy_stack_global.vi" "X-Minimum"() -> (w1379:dbl)
                  n822 = global read "xy_stack_global.vi" "Y-Minimum"() -> (w1378:dbl)
                  n823 = Increment(x=w1381) -> (x+1=w1380:u16)
                  n824 = local write "# steps"(w1380) -> ()
                  n825 = Add(x=w1382, y=w1383) -> (x+y=w1377:dbl)
                }
              }
              n826 = And(x=w1358, y=w1363) -> (x .and. y?=w1362:bool)
              n827 = local read "z-Stacking"() -> (w1323:bool)
              n828 = global write "xy_stack_global.vi" "requested x-position"(w1337) -> ()
              n829 = global write "xy_stack_global.vi" "requested y-position"(w1326) -> ()
              n830 = local write "requested z-Position"(w1342) -> ()
              n831 = local read "xy-Stacking"() -> (w1330:bool)
              n832 = local read "z-Stacking"() -> (w1331:bool)
              n833 = local read "z-Maximum"() -> (w1364:dbl)
              n834 = local read "Scan no."() -> (w1343:i32)
              n835 = Not(x=w1323) -> (.not. x?=w1322:bool)
              n836 = local read "Scan"() -> (w1339:bool)
              n837 = Not Or(1:w1331, 2:w1330) -> (0:w1329:bool)
              n838 = And(x=w1322, y=w1325) -> (x .and. y?=w1324:bool)
              n839 = Not(x=w1339) -> (.not. x?=w1327:bool)
              n840 = Greater?(x=w1342, y=w1364) -> (0:w1361:bool)
              n841 = Unbundle By Name(w1356) -> ("status"=w1328:bool)
              n842 = Compound Arithmetic op=OR(w1328, w1327, w1324, w1329, w1361) -> (w1360:bool)
              n843 = case shown="True" w1362 {
                tunnel: w1359 -> [_ w1392]
                tunnel: w1360 -> [_ w1390]
                tunnel: w1343 -> [_ w1385]
                tunnel: w1357 -> [_ w1389]
                tunnel: w1355 -> [_ w1387]
                tunnel: w1354 -> [_ w1384]
                frame False {
                }
                frame True {
                  n844 = local read "Detector"() -> (w1386:u16)
                  n845 = local read "Info File contents"() -> (w1393:string)
                  n846 = local read "Additional info"() -> (w1395:string)
                  n847 = Concatenate Strings("info: " ("string"), w1395, "\n", w1393) -> (w1391:string)
                  n848 = local read "Path"() -> (w1388:path)
                  n849 = case shown="1" w1386 {
                    tunnel: w1388 -> [_ w1407 w1418]
                    tunnel: w1387 -> [_ w1405 _]
                    tunnel: w1385 -> [_ w1401 w1414]
                    tunnel: w1384 -> [_ _ w1411]
                    frame 0, Default {
                    }
                    frame 1 {
                      n850 = local read "requested z-Position"() -> (w1398:dbl)
                      n851 = Path To String(path=w1407) -> (string=w1403:string)
                      n852 = Number To Decimal String(number=w1401) -> (decimal integer string=w1404:string)  [unwired: 1 in]
                      n853 = Number To Decimal String(number=w1398) -> (decimal integer string=w1397:string)  [unwired: 1 in]
                      n854 = Concatenate Strings(w1403, "_" ("string"), w1404, "_" ("string"), w1397, "_um_spectrum.dat" ("string")) -> (w1410:string)
                      n855 = String To Path(string=w1410) -> (path=w1406:path)
                      n856 = Write to Binary File(file (use dialog)=w1406, data=w1405) -> (refnum out=w1408:refnum<file>, error out=w1409:errorcluster)  [unwired: 4 in, 1 out]
                      n857 = Close File(refnum=w1408, error in=w1409) -> ()  [unwired: 2 out]
                    }
                    frame 2 {
                      n858 = Path To String(path=w1418) -> (string=w1413:string)
                      n859 = Number To Decimal String(number=w1414) -> (decimal integer string=w1415:string)  [unwired: 1 in]
                      n860 = Concatenate Strings(w1413, "_" ("string"), w1415, "_OCM.dat" ("string")) -> (w1421:string)
                      n861 = String To Path(string=w1421) -> (path=w1417:path)
                      n862 = Write to Binary File(file (use dialog)=w1417, data=w1411) -> (refnum out=w1419:refnum<file>, error out=w1420:errorcluster)  [unwired: 4 in, 1 out]
                      n863 = Close File(refnum=w1419, error in=w1420) -> ()  [unwired: 2 out]
                    }
                  }
                  n864 = call "save_to_disk.vi"("Retrace"=w1389, "slice"=w1385, "write info file?"=w1390, "Scan info"=w1391, "Image"=w1392, "File path"=w1388) -> ()  [unwired: 3 in, 1 out]
                }
              }
              "Retrace" <- w1357
              "spectral image" <- w1355
              "OCM Array" <- w1354
            }
          }
          n865 = local read "z-Stacking"() -> (w746:bool)
        }
      }
      frame #5 {
        w1435 = path "C:/Data/scan.log" ("path to log")
        # "The device is cleared, the cursors are moved to the image edge.\nThe log-file is updated."
        n866 = local read "xy-Stacking"() -> (w1422:bool)
        n867 = case shown="False" w1430 {
          tunnel: w1435 -> [w1448 w1453]
          frame False {
            n868 = Get Date/Time In Seconds() -> (seconds since 1Jan1904=w1446:timestamp)
            n869 = Format Into String(format string="%T: Scan stopped\\n", w1446) -> (resulting string=w1445:string)  [unwired: 2 in, 1 out]
            n870 = call <vilib>:"Write Characters To File.vi"("append to file? (new file:F)"=TRUE, "character string"=w1445, "file path (dialog if empty)"=w1448) -> ()  [unwired: 2 in, 1 out]
          }
          frame True {
            n871 = Get Date/Time In Seconds() -> (seconds since 1Jan1904=w1451:timestamp)
            n872 = Format Into String(format string="%<%Y-%m-%d %H:%M:%S>T: Slice scan finished\\n", w1451) -> (resulting string=w1450:string)  [unwired: 2 in, 1 out]
            n873 = call <vilib>:"Write Characters To File.vi"("append to file? (new file:F)"=TRUE, "character string"=w1450, "file path (dialog if empty)"=w1453) -> ()  [unwired: 2 in, 1 out]
          }
        }
        n874 = Unbundle By Name(w1427) -> ("status"=w1432:bool, "code"=w1433:i32, "source"=w1434:string)
        n875 = case shown="True" w1422 {
          frame False {
          }
          frame True {
            # "reset x and y minima"
            n876 = global read "xy_stack_global.vi" "X-Minimum"() -> (w1437:dbl)
            n877 = global read "xy_stack_global.vi" "Y-Minimum"() -> (w1436:dbl)
            n878 = global write "xy_stack_global.vi" "requested x-position"(w1437) -> ()
            n879 = global write "xy_stack_global.vi" "requested y-position"(w1436) -> ()
          }
        }
        n880 = case shown="False" w1432 {
          tunnel: w1433 -> [_ w1439]
          tunnel: w1434 -> [_ w1438]
          tunnel: w1435 -> [_ w1443]
          frame False {
          }
          frame True {
            n881 = Get Date/Time In Seconds() -> (seconds since 1Jan1904=w1440:timestamp)
            n882 = Format Into String(format string="%<%Y-%m-%d %H:%M:%S>T: Error encountered: %d: %s. Scan will abort.\\n", w1440, w1439, w1438) -> (resulting string=w1441:string)  [unwired: 2 in, 1 out]
            n883 = call <vilib>:"Write Characters To File.vi"("append to file? (new file:F)"=TRUE, "character string"=w1441, "file path (dialog if empty)"=w1443) -> ()  [unwired: 2 in, 1 out]
          }
        }
        n884 = local read "write task"() -> (w1424:refnum<k21>)
        n885 = local read "read task"() -> (w1423:refnum<k21>)
        n886 = call <vilib>:"DAQmx Clear Task.vi"("task in"=w1424) -> ("error out"=w1426:errorcluster)  [unwired: 14 in]
        n887 = call <vilib>:"DAQmx Clear Task.vi"("task in"=w1423) -> ("error out"=w1425:errorcluster)  [unwired: 14 in]
        n888 = Merge Errors(w1427, w1426, w1425) -> (w1428:errorcluster)
        n889 = Unbundle By Name(w1428) -> ("status"=w1431:bool)
        n890 = local write "System"(w1431) -> ()
        n891 = local write "Scan"(FALSE ("Scan")) -> ()
      }
    }
  }
  n892 = call <vilib>:"Simple Error Handler.vi"("error in (no error)"=w21) -> ()  [unwired: 4 in, 5 out]
